vi "Main.vi"() -> ()   [LabVIEW 2013]
doc: "This Continuous Measurement sample project is based on the Queued Message Handler template.\n\nThe Event Handling Loop generates messages based on user interface actions.\n\nThe Message Handling Loop processes messages generated by the Event Handling Loop, or by other messages. There are also Acquisition and Logging message handling loop subVIs, and a chart updating loop."
uses:
  Settings/Settings.ctl
  Logging/Logging Configuration.ctl
  Piezo/Hardware Configuration.ctl
  Capacitive/Hardware Configuration.ctl
  Acquisition/Hardware Configuration.ctl
  Acquisition/Counter Configuration.ctl
  ADC/ADC Configuration.ctl
  controls/UI Data.ctl
  controls/UI State.ctl
  support/Message Queue/Enqueue Message (Single).vi
  <vilib>/measure/madcrms.llb/Averaged DC-RMS for 1 Chan.vi
  <vilib>/Utility/error.llb/Error Cluster From Error Code.vi
  <vilib>/ErrorRing/Error Ring.xnode
  Acquisition/Acquisition.lvlib
  Logging/Logging.lvlib
  Settings/Settings.lvlib
  support/User Event - Stop/User Event - Stop.lvlib
  support/Message Queue/Message Queue.lvlib
  <vilib>/ptbypt/NI_PtbyPt.lvlib
  Piezo/Piezo.lvlib
  Feedback/Feedback.lvlib
  <vilib>/measure/NI_MAPro.lvlib
  XY/XY.lvlib
  support/Data Notifiers/Data Notifiers.lvlib
  Capacitive/Capacitive.lvlib
  Automation/Automation.lvlib
panel:
  in  "Max. Samp":i32=1000000 format="%^#.2e"
  in  "Abort":bool
  out "Auto Status":string
  out "Status 2":bool
  out "Waveform Chart 2":dbl(graph)
  out "mean":dbl format="%0.2f"
  out "Error":dbl(knob) scale=-300.0..300.0
  in  "Channel":i32(ring) items=["0", "1", "2", "3", "off"]
  in  "Red":i32(ring) items=["0", "1", "2", "3", "off"]
  in  "Blue":i32(ring) items=["0", "1", "2", "3", "off"]
  out "Sample Rate (s/s)":i32
  out "Waveform Chart":waveform(dbl)[](graph)
  in  "Start Z scan":bool
  in  "Enable Piezo":bool
  out "Path":path
  in  "Filename":string
  out "Data Source":string="Counter (APD)"
  in  "Feedback Settings":T1={"Setpoint (cnt)"=10.999878508704048, "Refresh Time (s)"=1.0, "K_p (nm/cnt)"=50.0, "Averaging Time"=1.0, "T_i (s)"=0.3, "T_d (s)"=1.0, "Error Signal Source"=1} {"Error Signal Source" items=["APD Signal", "Capacitive"]}
  in  "Scan!":bool
  in  "Auto \nFB On":bool
  out "Control Status":string
  in  "Averaging Time (s)":dbl=3.0
  in  "Average and send\nto Setpoint":bool
  out "average":dbl
  out "Cap Readout":sgl
  out "Cap Status":string
  in  "Enable Sensor":bool
  out "Status 4":string
  in  "initialize":bool
  in  "PSD points":i32=1000
  out "Status 3":string
  out "Y":sgl
  out "X":sgl
  in  "Next Button":bool
  in  "Up Button":bool
  in  "Down Button":bool
  in  "Previous Button":bool
  in  "Jog Speed":u16(ring) items=["0", "1", "2", "3"]
  in  "Enable XY":bool
  out "Status":bool
  in  "Enable Feedback!":bool
  in  "Scan Settings":T2={"Dwell Time (s)"=1.0, "Max Height"=10.0, "Min Height"=9.0, "Step Size (um)"=0.01}
  in  "Start Saving":bool
  out "PiezoPosition":sgl
  out "Scan Duration: (s)":dbl
  in  "Do move":bool
  in  "Move to (um)":sgl
  out "PSD":cluster{"t":dbl, dbl, "Power Spectrum":dbl[]}(graph)
  out "Data":waveform(dbl)[](graph)
  in  "Settings":bool
  in  "Start":bool
  in  "Stop":bool
  out "Status":string
  in  "Exit":bool
  # "Recording"
  # "Position Control"
  # "Acquisition"
  # "Automation"
  # "Piezo Controller"
  # "X-Y Stage"
  # "Displacement Sensor"
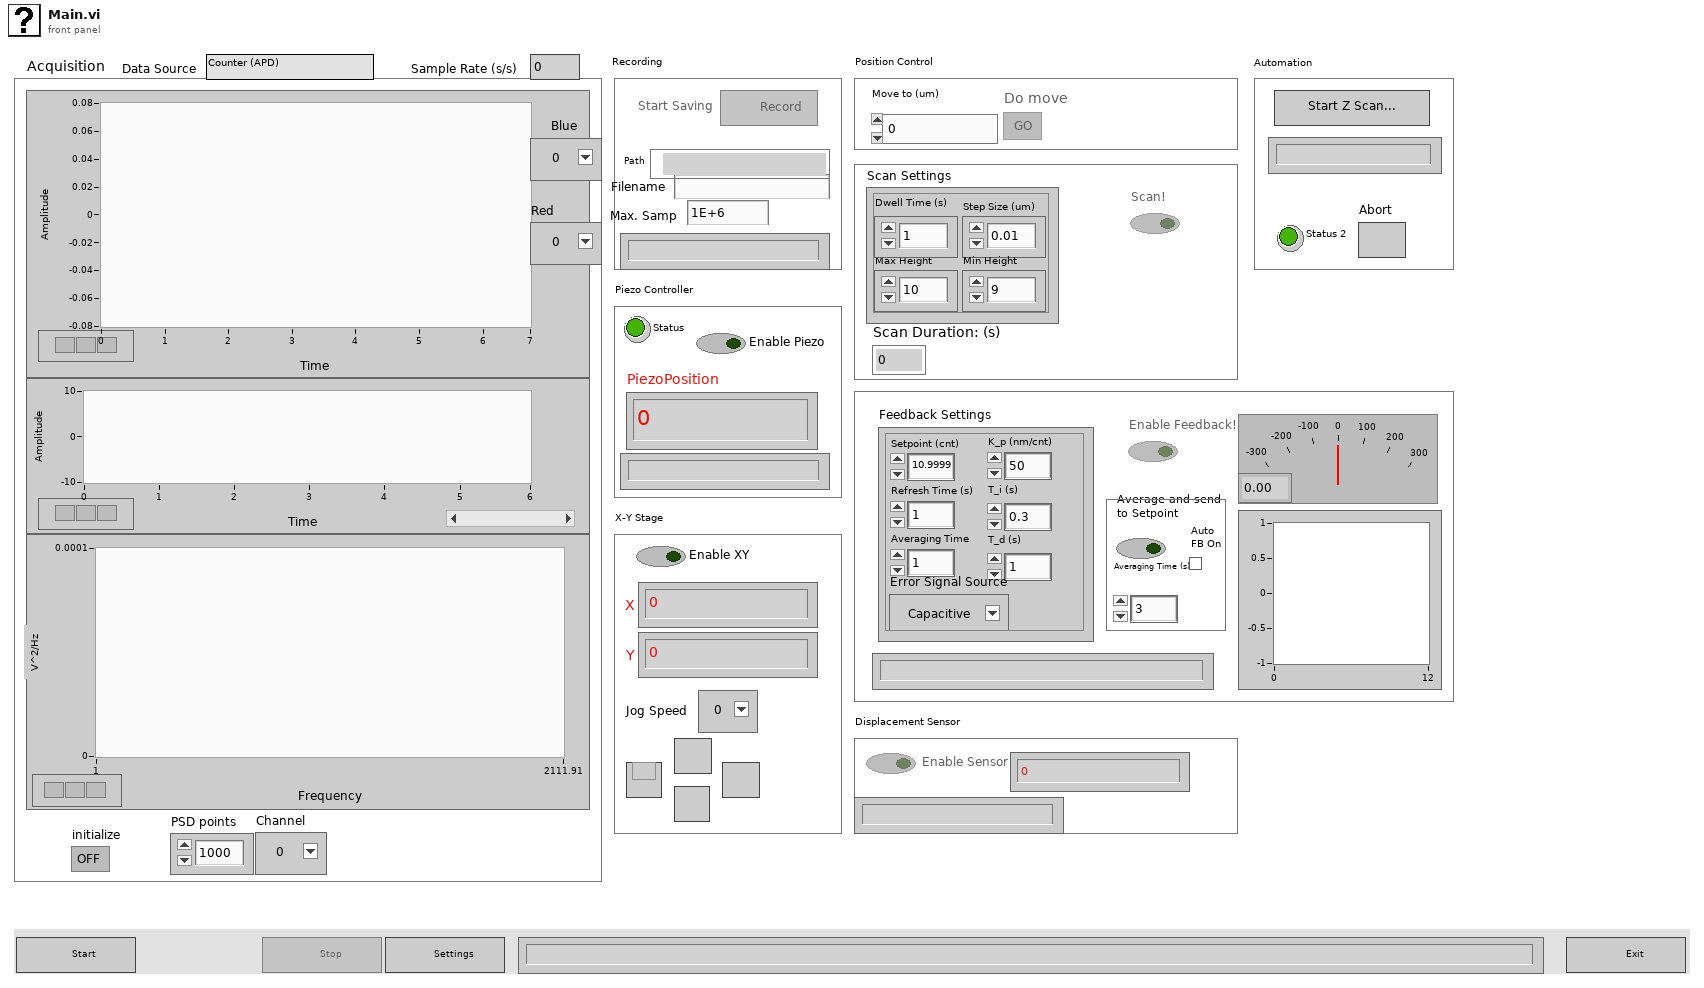
[diagram p1: front panel]
types:
  T1 = cluster{"Setpoint (cnt)":dbl, "Refresh Time (s)":dbl, "K_p (nm/cnt)":dbl, "Averaging Time":dbl, "T_i (s)":dbl, "T_d (s)":dbl, "Error Signal Source":u16}
  T2 = cluster{"Dwell Time (s)":dbl, "Max Height":dbl, "Min Height":dbl, "Step Size (um)":dbl}
  T3 = typedef "UI State.ctl" = cluster{"UI State":enum16{"Idle", "Acquiring and Logging", "Waiting for Exit", "Waiting for Stop"}, "Acq On":bool, "Log On":bool, "Piezo On":bool, "XY On":bool, "Cap On":bool}
  T4 = typedef "UI Data.ctl" = cluster{"Start Ref":refnum<vi>, "Trigger Ref":refnum<vi>, "Stop Ref":refnum<vi>, "Settings Ref":refnum<vi>, "Status Ref":refnum<vi>, "Exit Ref":refnum<vi>, "Data Ref":refnum<vi>, "Record Ref":refnum<vi>, "Scan Ref":refnum<vi>, "Feedback Ref":refnum<vi>, "Enable Sensor Ref":refnum<vi>, "Enable XY Ref":refnum<vi>, "Do move ref":refnum<vi>, "Enable Piezo":refnum<vi>}
  T5 = typedef "Settings.lvlib/Settings.ctl" = cluster{"Logging Configuration":T6, "Piezo Config":T7, "Capacitive Config":T8, "Hardware Config":T9}
  T6 = typedef "Logging.lvlib/Logging Configuration.ctl" = cluster{"Log File Base Path":path, "Max Samples":u32, "File Refnum":refnum<file>, "Log Piezo":bool, "Piezo File Refnum":refnum<file>, "Log Capacitive":bool, "Cap File Refnum":refnum<file>, "Filename":string, "Path where to save":path}
  T7 = typedef "Piezo.lvlib/Hardware Configuration.ctl" = cluster{"Piezo Serial Number":i32, "MG17Piezo":refnum<k7>, "Setpoint (um)":sgl}
  T8 = typedef "Capacitive.lvlib/Hardware Configuration.ctl" = cluster{"IP Address":string, "Handle":u32, "Refresh Time (ms)":dbl}
  T9 = typedef "Acquisition.lvlib/Hardware Configuration.ctl" = cluster{"Data Source":u16, "Counter Configuration":T10, "ADC Configuration":T11}
  T10 = typedef "Acquisition.lvlib/Counter Configuration.ctl" = cluster{"DAQmx Task":refnum<k21>, "Counter(s)":tag, "samples per readout":i32}
  T11 = typedef "Acquisition.lvlib/ADC Configuration.ctl" = cluster{"DAQmx Task":refnum<k21>, "Channel(s)":tag, "samples per readout":i32, "Sample Rate (s/s)":i32, "Max Voltage":dbl, "Min Voltage":dbl}
  T12 = typedef "Data Notifiers.lvlib/All Data Notifiers.ctl" = cluster{"APD Data Notifier":refnum<notifier>, "Piezo Readout Notifier":refnum<notifier>, "XY Readout Notifier":refnum<notifier>, "Capacitive Readout Notifier":refnum<notifier>, "Error Signal Notifier":refnum<notifier>}
  T13 = typedef "Message Queue.lvlib/All Message Queues.ctl" = cluster{"UI":refnum<queue>, "Acquisition":refnum<queue>, "Logging":refnum<queue>, "Piezo":refnum<queue>, "Feedback":refnum<queue>, "XY":refnum<queue>, "Capacitive":refnum<queue>, "Automation":refnum<queue>}
  T14 = enum16{"Idle", "Acquiring and Logging", "Waiting for Exit", "Waiting for Stop"}
  T15 = enum8{"Enabled", "Disabled", "Disabled and Grayed Out"}
  T16 = cluster{"Averaging Time (s)\n":dbl, "Error Signal Source":u16}
  T17 = cluster{"Value":bool, "Filename":string, "Max. Samp":i32}
  T18 = typedef "Automation.lvlib/Zscan Settings.ctl" = cluster{"Heights":dbl[], "Seconds per height":i32, "First Data Index":i32}
  T19 = typedef "XY.lvlib/XY Display.ctl" = cluster{"X Position":sgl, "Y Position":sgl}
  T20 = typedef "Acquisition.lvlib/APD Notifier Cluster.ctl" = cluster{"data":dbl[][], "t0":i32}
  T21 = typedef "Piezo.lvlib/Piezo display.ctl" = cluster{"PiezoPosition":sgl, "Counter Time":i32}
  T22 = typedef "Control 3.ctl" = cluster{"Error signal":dbl[], "Setpoint":dbl, "Last average":dbl}
  T23 = typedef "Capacitive.lvlib/Capacitive Signal Cluster.ctl" = cluster{"Readout":sgl, "Time":i32, "Temperature":dbl}
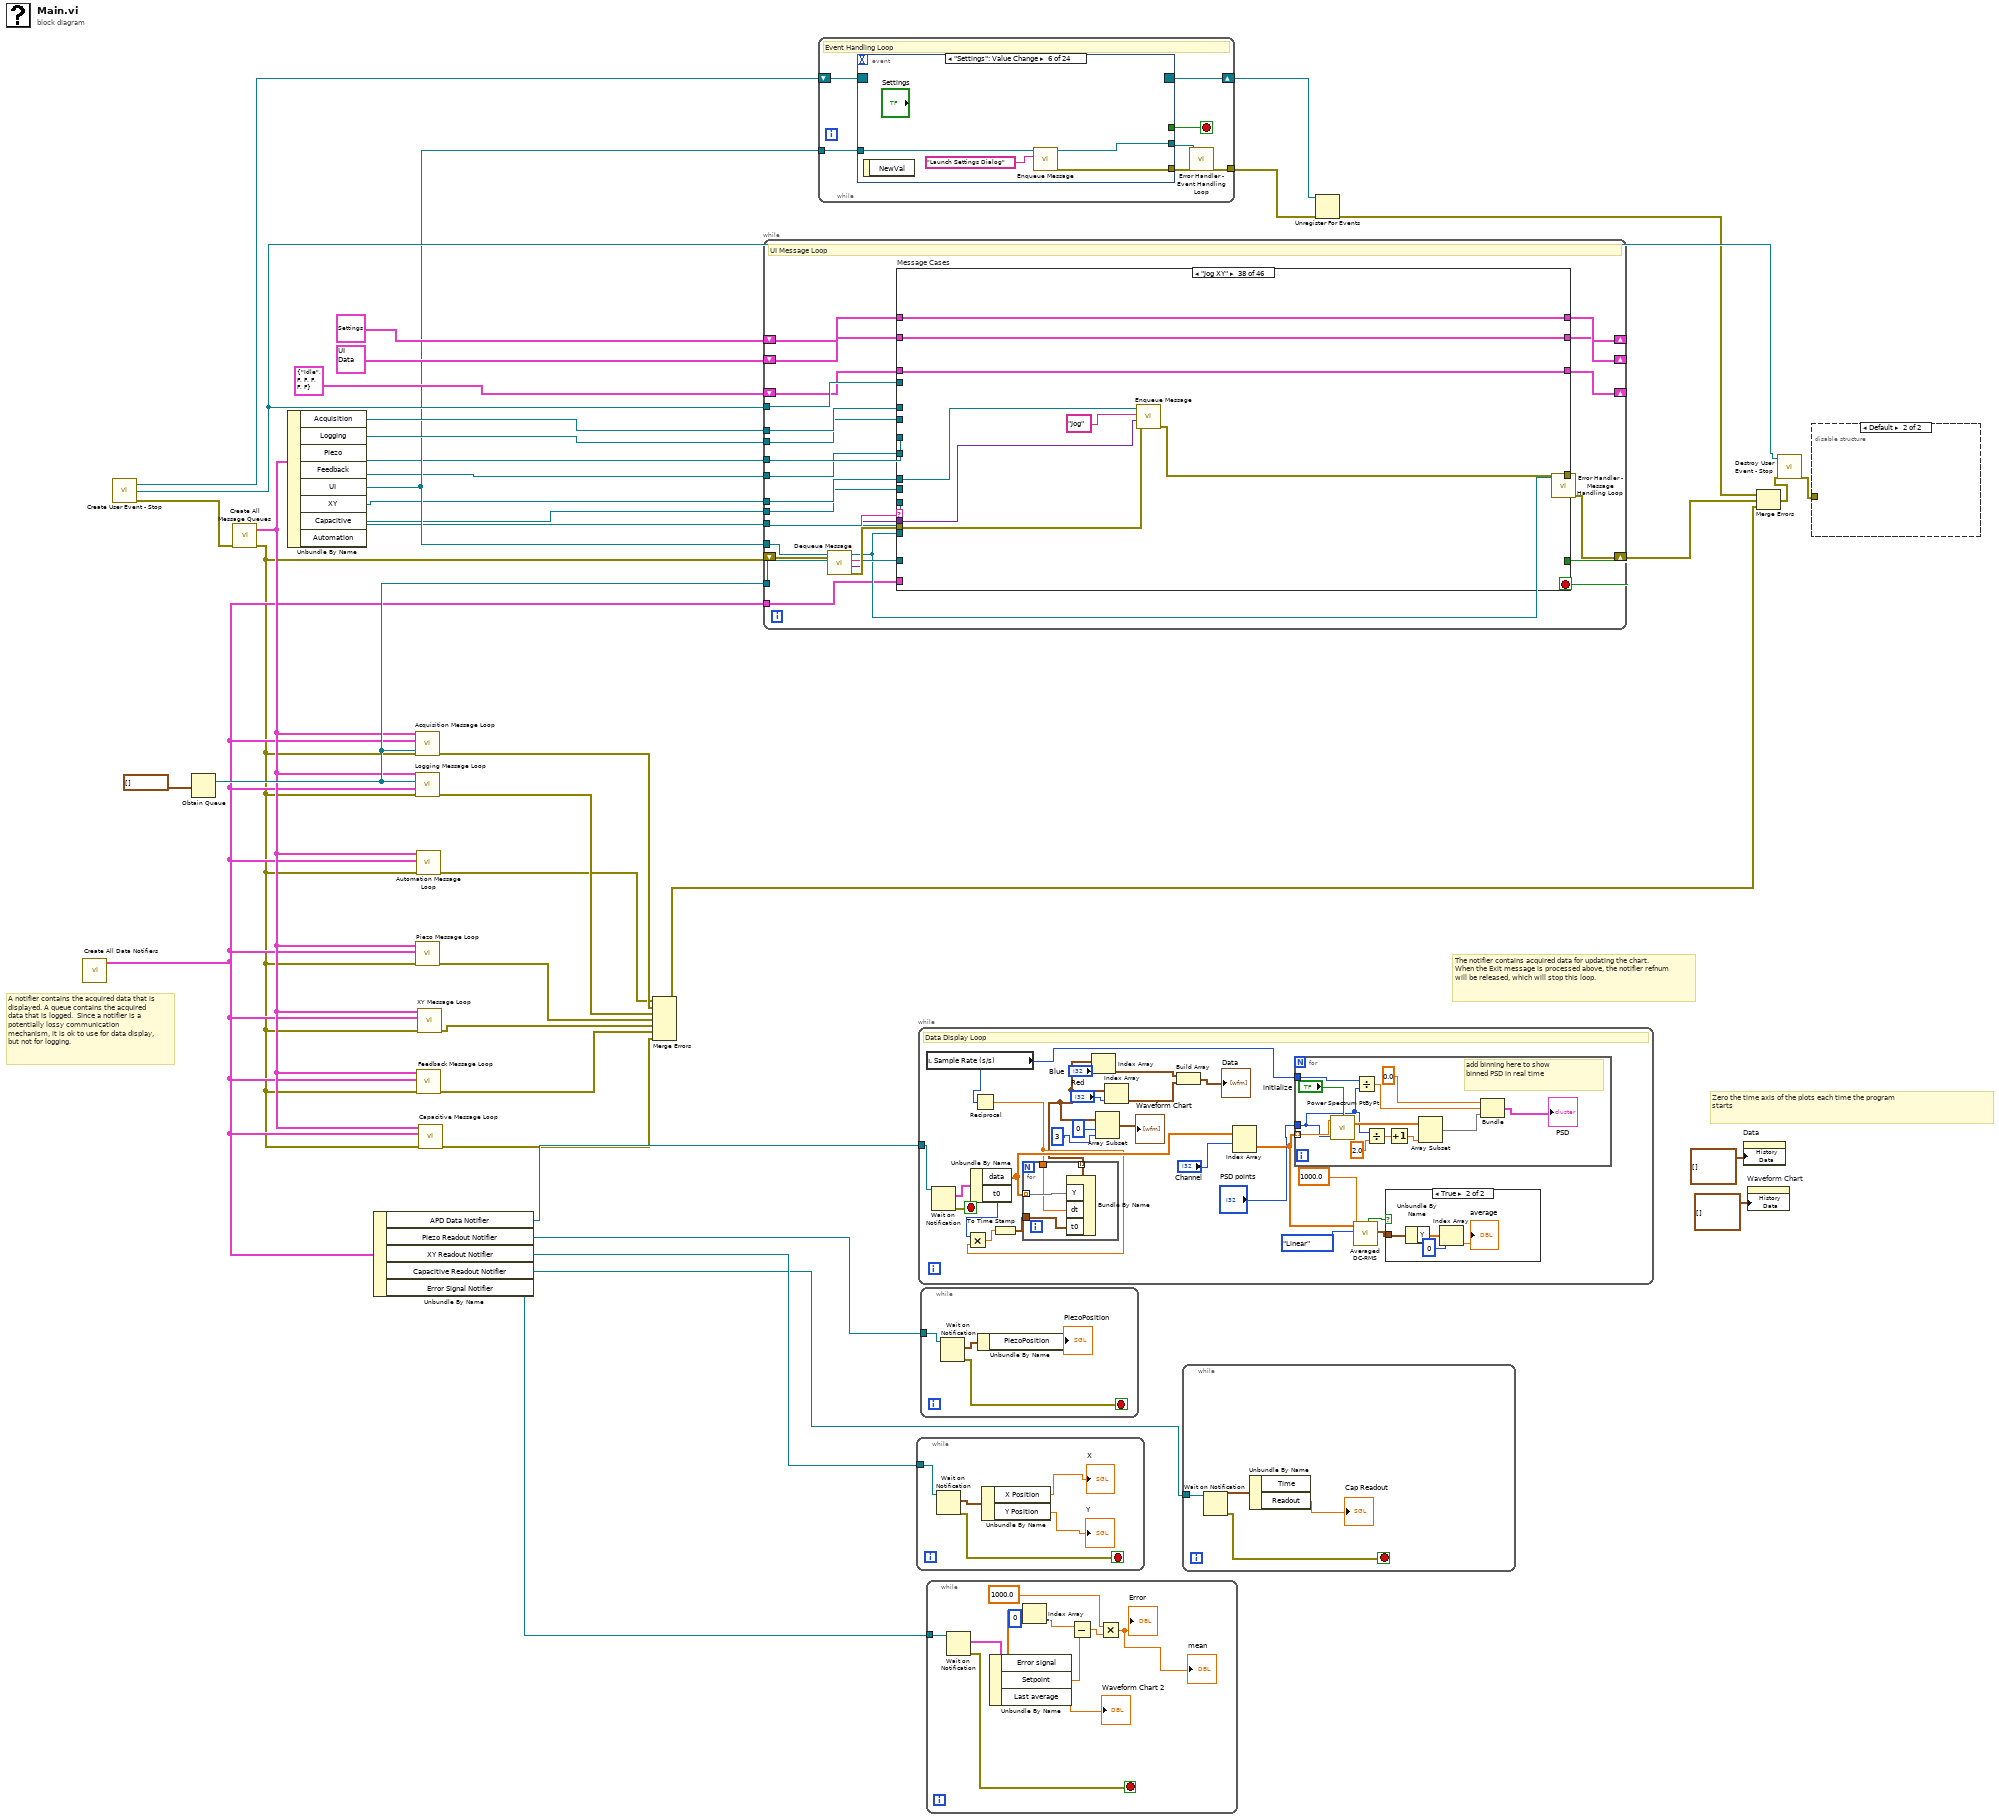
[diagram p0: block diagram]
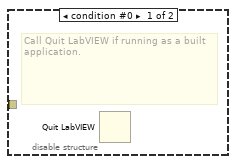
[diagram p2: hidden frame]
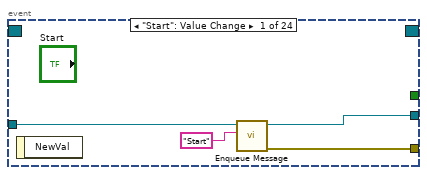
[diagram p4: hidden frame]
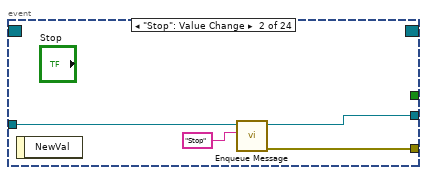
[diagram p5: hidden frame]
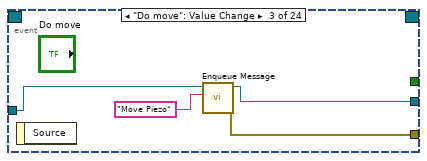
[diagram p6: hidden frame]
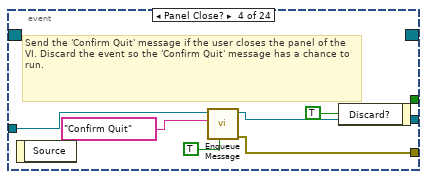
[diagram p7: hidden frame]
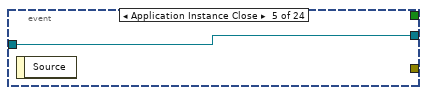
[diagram p8: hidden frame]
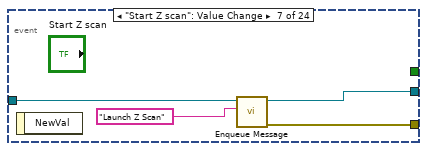
[diagram p9: hidden frame]
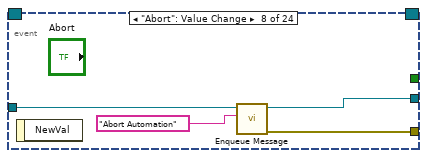
[diagram p10: hidden frame]
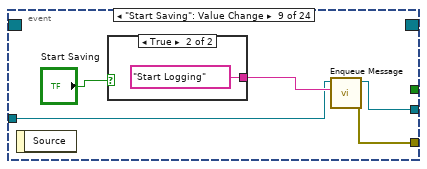
[diagram p11: hidden frame]
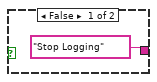
[diagram p12: hidden frame]
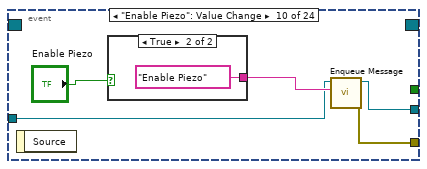
[diagram p13: hidden frame]
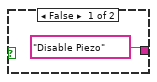
[diagram p14: hidden frame]
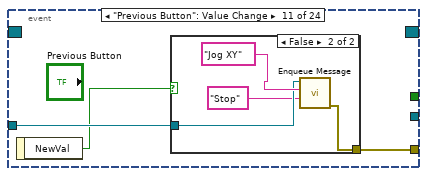
[diagram p15: hidden frame]
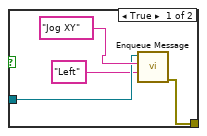
[diagram p16: hidden frame]
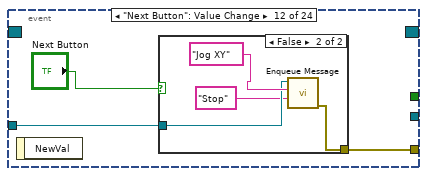
[diagram p17: hidden frame]
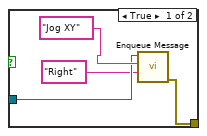
[diagram p18: hidden frame]
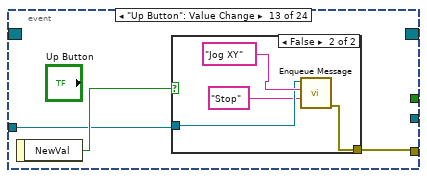
[diagram p19: hidden frame]
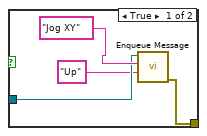
[diagram p20: hidden frame]
diagram:
  # "Zero the time axis of the plots each time the program \nstarts"
  # "A notifier contains the acquired data that is displayed. A queue contains the acquired data that is logged.  Since a notifier is a potentially lossy communication mechanism, it is ok to use for data display, but not for logging."
  # "The notifier contains acquired data for updating the chart. When the Exit message is processed above, the notifier refnum will be released, which will stop this loop."
  n1 = call "Create All Data Notifiers.vi"() -> ("Initialized Data Notifiers"=w3:T12)  [unwired: 11 in]
  n2 = call "Create User Event - Stop.vi"() -> ("error out"=w35:errorcluster, "User Event - Stop"=w36:refnum<user-event>, "Stop Event Registration Refnum"=w37:refnum<event-registration>)  [unwired: 9 in]
  n3 = Obtain Queue(element data type=waveform(dbl)[] []) -> (queue out=w27:refnum<queue>)  [unwired: 4 in, 2 out]
  n4 = call "Create All Message Queues.vi"("error in (no error)"=w35) -> ("error out"=w2:errorcluster, "Message Queues out"=w4:T13)  [unwired: 9 in]
  n5 = Unbundle By Name(w4) -> ("Acquisition"=w30:refnum<queue>, "Logging"=w29:refnum<queue>, "Piezo"=w23:refnum<queue>, "Feedback"=w22:refnum<queue>, "UI"=w24:refnum<queue>, "XY"=w21:refnum<queue>, "Capacitive"=w17:refnum<queue>, "Automation"=w5:refnum<queue>)
  n6 = Unbundle By Name(w3) -> ("APD Data Notifier"=w20:refnum<notifier>, "Piezo Readout Notifier"=w19:refnum<notifier>, "XY Readout Notifier"=w18:refnum<notifier>, "Capacitive Readout Notifier"=w9:refnum<notifier>, "Error Signal Notifier"=w6:refnum<notifier>)
  n7 = call "Acquisition Message Loop.vi"("error in (no error)"=w2, "Data Queue"=w27, "Data Notifiers"=w3, "Message Queues"=w4) -> ("error out"=w13:errorcluster)  [unwired: 7 in]
  n8 = call "Logging Message Loop.vi"("error in (no error)"=w2, "Data Notifiers"=w3, "Data Queue"=w27, "Message Queues"=w4) -> ("error out"=w14:errorcluster)  [unwired: 7 in]
  n9 = call "Piezo Message Loop.vi"("error in (no error)"=w2, "Data Notifiers"=w3, "Message Queues"=w4) -> ("error out"=w15:errorcluster)  [unwired: 8 in]
  n10 = call "Automation Message Loop.vi"("error in (no error)"=w2, "Data Notifiers"=w3, "Message Queues"=w4) -> ("error out"=w1:errorcluster)  [unwired: 8 in]
  n11 = call "Feedback Message Loop.vi"("error in (no error)"=w2, "Data Notifiers"=w3, "Message Queues"=w4) -> ("error out"=w12:errorcluster)  [unwired: 8 in]
  n12 = call "XY Message Loop.vi"("error in (no error)"=w2, "Data Notifiers"=w3, "Message Queues"=w4) -> ("error out"=w16:errorcluster)  [unwired: 8 in]
  n13 = call "Capacitive Message Loop.vi"("error in (no error)"=w2, "Data Notifiers"=w3, "Message Queues"=w4) -> ("error out"=w11:errorcluster)  [unwired: 8 in]
  n14 = Merge Errors(w1, w13, w14, w15, w16, w12, w11) -> (w10:errorcluster)
  n15 = while {
    tunnel: w24 -> [w59]
    tunnel: w36 -> [w64]
    shift-right: [w50] -> w40
    shift-left: w2 -> [w63]
    shift-right: [w58] -> _
    shift-left: T5 {"Logging Configuration"={"Log File Base Path"=path "", "Max Samples"=0, "File Refnum"=refnum, "Log Piezo"=FALSE, "Piezo File Refnum"=refnum, "Log Capacitive"=FALSE, "Cap File Refnum"=refnum, "Filename"="", "Path where to save"=path ""}, "Piezo Config"={"Piezo Serial Number"=0, "MG17Piezo"=refnum, "Setpoint (um)"=0.0}, "Capacitive Config"={"IP Address"="", "Handle"=0, "Refresh Time (ms)"=0.0}, "Hardware Config"={"Data Source"=0, "Counter Configuration"={"DAQmx Task"="", "Counter(s)"="", "samples per readout"=0}, "ADC Configuration"={"DAQmx Task"="", "Channel(s)"="", "samples per readout"=0, "Sample Rate (s/s)"=0, "Max Voltage"=0.0, "Min Voltage"=0.0}}} ("Settings") -> [w57]
    shift-right: [w55] -> _
    shift-left: T4 {"Start Ref"=refnum, "Trigger Ref"=refnum, "Stop Ref"=refnum, "Settings Ref"=refnum, "Status Ref"=refnum, "Exit Ref"=refnum, "Data Ref"=refnum, "Record Ref"=refnum, "Scan Ref"=refnum, "Feedback Ref"=refnum, "Enable Sensor Ref"=refnum, "Enable XY Ref"=refnum, "Do move ref"=refnum, "Enable Piezo"=refnum} ("Measurement UI Controls") -> [w56]
    tunnel: w30 -> [w54]
    tunnel: w29 -> [w53]
    tunnel: w27 -> [w52]
    shift-right: [w47] -> _
    shift-left: T3 {"UI State"=enum."Idle", "Acq On"=FALSE, "Log On"=FALSE, "Piezo On"=FALSE, "XY On"=FALSE, "Cap On"=FALSE} ("UI State") -> [w48]
    tunnel: w23 -> [w46]
    tunnel: w22 -> [w45]
    tunnel: w21 -> [w44]
    tunnel: w3 -> [w43]
    tunnel: w17 -> [w42]
    tunnel: w5 -> [w41]
    stop <- w65 stop-if-true
    # "UI Message Loop"
    n16 = call "Dequeue Message.vi"("error in (no error)"=w63, "Message Queue"=w59) -> ("error out"=w62:errorcluster, "Message Data"=w60:variant, "Message"=w61:string, "dup Message Queue"=w49:refnum<queue>)  [unwired: 6 in]
    n17 = case "Message Cases" shown="\"Jog XY\"" w61 {
      selector: w61 -> [_ _ _ _ _ _ _ _ _ _ _ _ _ _ _ _ _ _ _ _ _ _ _ _ _ _ _ _ _ _ _ _ _ _ _ _ _ _ _ _ _ _ _ _ _ w807]
      tunnel: w49 -> [w70 _ _ _ _ _ _ _ w282 w317 w329 w351 w369 w388 w411 _ w455 w470 w482 w520 _ _ _ _ _ _ _ _ _ _ _ _ _ _ _ _ _ _ _ _ _ _ _ w773 w793 _]
      tunnel: w62 -> [w69 w103 w114 w128 w139 w153 w167 w186 w281 w316 w327 w349 w367 w386 w410 w444 w457 w474 w481 w525 w535 w540 w547 w555 w567 w574 w589 w605 w613 w624 w640 w649 w665 w672 w680 w696 w707 w713 w722 w730 w738 w750 w761 w775 w795 _]
      tunnel: [w76 w103 w115 w129 w140 w154 w168 w187 w283 w304 w328 w350 w368 w387 w407 w447 w452 w465 w480 w526 w534 w539 w553 w561 w566 w580 w583 w611 w619 w630 w644 w655 w669 w677 w686 w700 w711 w712 w721 w735 w743 w754 w765 w776 w796 w808] -> w51
      tunnel: [_ _ _ _ _ _ _ _ _ _ _ _ _ _ _ _ _ _ _ TRUE _ _ _ _ _ _ _ _ _ _ _ _ _ _ _ _ _ _ _ _ _ _ _ _ _ _] -> w65
      tunnel: w60 -> [_ _ w113 w127 w138 w152 w166 w185 _ _ _ _ _ _ _ _ _ w473 _ _ _ _ _ _ _ _ w588 _ _ w631 _ _ _ _ _ _ _ w716 w723 _ _ _ _ _ _ _]
      tunnel: w64 -> [_ _ _ _ _ _ _ _ _ _ _ _ _ _ _ _ _ _ _ w524 _ _ _ _ _ _ _ _ _ _ _ _ _ _ _ _ _ _ _ _ _ _ _ _ _ _]
      tunnel: [w79 w102 w110 w124 w135 w149 w163 w183 w280 w315 w335 w356 w375 w394 w417 w431 w454 w476 w484 w522 w533 w543 w552 w560 w572 w579 w592 w610 w618 w634 w643 w654 w668 w676 w685 w699 w710 w719 w727 w734 w742 w753 w764 w778 w798 w810] -> w58
      tunnel: w57 -> [w80 w102 w110 w124 w135 w149 w163 w183 w280 w315 w335 w356 w375 w394 w417 w431 w458 w476 w484 w522 w533 w543 w552 w560 w572 w579 w592 w610 w618 w634 w643 w654 w668 w676 w685 w699 w710 w719 w727 w734 w742 w753 w764 w778 w798 w810]
      tunnel: w56 -> [w72 w101 w109 w123 w131 w145 w162 w182 w262 w297 w334 w348 w374 w393 w416 w443 w451 w475 w483 w521 w532 w542 w551 w559 w571 w578 w591 w609 w617 w633 w636 w651 w663 w675 w684 w692 w703 w718 w726 w733 w741 w747 w758 w777 w797 w809]
      tunnel: [w72 w100 w109 w123 w131 w145 w162 w182 w262 w297 w334 w348 w374 w393 w416 w443 w451 w475 w483 w521 w532 w542 w551 w559 w571 w578 w591 w609 w617 w633 w636 w651 w663 w675 w684 w692 w703 w718 w726 w733 w741 w747 w758 w777 w797 w809] -> w55
      tunnel: w54 -> [_ _ _ _ _ _ _ _ w273 w293 _ _ _ _ _ w442 _ _ _ w513 _ _ _ _ _ _ _ _ _ _ _ _ _ _ _ _ _ _ _ _ _ _ _ _ _ _]
      tunnel: w53 -> [_ _ _ _ _ _ _ _ _ w292 _ _ _ _ _ w441 _ _ _ w512 _ _ _ _ _ _ _ w606 w614 _ _ _ _ _ _ _ _ _ _ _ _ _ _ _ _ _]
      tunnel: w52 -> [_ _ _ _ _ _ _ _ _ _ _ _ _ _ _ _ _ _ _ w519 _ _ _ _ _ _ _ _ _ _ _ _ _ _ _ _ _ _ _ _ _ _ _ _ _ _]
      tunnel: w48 -> [_ _ w104 w121 w134 w148 w161 w181 _ w305 w332 w354 w372 w391 w414 w440 w450 w464 w478 _ w531 w536 w550 w558 w570 w577 w590 w608 w616 w623 w642 w653 w667 w674 w683 w698 w709 w714 w720 w732 w740 w752 w763 w774 w794 w806]
      tunnel: [T3 {"UI State"=enum."Idle", "Acq On"=FALSE, "Log On"=FALSE, "Piezo On"=FALSE, "XY On"=FALSE, "Cap On"=FALSE} ("UI State") T3 {"UI State"=enum."Idle", "Acq On"=FALSE, "Log On"=FALSE, "Piezo On"=FALSE, "XY On"=FALSE, "Cap On"=FALSE} ("UI State") w104 w121 w134 w148 w161 w181 T3 {"UI State"=enum."Idle", "Acq On"=TRUE, "Log On"=TRUE, "Piezo On"=TRUE, "XY On"=FALSE, "Cap On"=FALSE} ("UI State") w307 w332 w354 w372 w391 w414 w440 w450 w464 w479 T3 {"UI State"=enum."Idle", "Acq On"=FALSE, "Log On"=FALSE, "Piezo On"=FALSE, "XY On"=FALSE, "Cap On"=FALSE} ("UI State") w531 w536 w550 w558 w570 w577 w590 w608 w616 w623 w642 w653 w667 w674 w683 w698 w709 w714 w720 w732 w740 w752 w763 w774 w794 w806] -> w47
      tunnel: w46 -> [_ _ _ _ _ _ _ _ w271 w291 _ _ _ _ _ _ _ _ _ w511 _ _ _ _ _ _ _ _ _ _ _ _ _ _ _ _ _ _ _ _ _ w748 w759 _ _ _]
      tunnel: w45 -> [_ _ _ _ _ _ _ _ w267 w290 _ _ _ _ _ _ _ _ _ w510 _ w538 w548 w556 w568 w575 _ _ _ _ w637 _ _ w670 w678 _ _ _ _ _ _ _ _ _ _ _]
      tunnel: w44 -> [_ _ _ _ _ _ _ _ _ w289 _ _ _ _ _ _ _ _ _ w509 _ _ _ _ _ _ _ _ _ _ _ _ _ _ _ w694 w705 w717 w724 _ _ _ _ _ _ _]
      tunnel: w43 -> [_ _ _ _ _ _ _ _ _ _ _ _ _ _ _ _ _ _ _ w516 _ _ _ _ _ _ _ _ _ _ _ _ _ _ _ _ _ _ _ _ _ _ _ _ _ _]
      tunnel: w42 -> [_ _ _ _ _ _ _ _ w264 w288 _ _ _ _ _ w439 _ _ _ w507 _ _ _ _ _ _ _ _ _ _ _ _ _ _ _ _ _ _ _ w728 w736 _ _ _ _ _]
      tunnel: w41 -> [_ _ _ _ _ _ _ _ _ w287 _ _ _ _ _ _ _ _ _ w506 _ _ _ _ _ _ _ _ _ _ _ w650 w662 _ _ _ _ _ _ _ _ _ _ _ _ _]
      frame "Initialize" {
        # "Initialize - Get configuration settings, then message the UI to initialize, and broadcast the settings to the other message loops."
        n18 = call "Load Settings from XML.vi"("Settings in"=w80) -> ("Settings out"=w79:T5)  [unwired: 9 in, 1 out]
        n19 = call-poly "Enqueue Message.vi"("error in (no error)"=w69, "Message"="Init UI Refs", "Message Queue"=w70) -> ("error out"=w67:errorcluster, "dup Message Queue"=w68:refnum<queue>)  [unwired: 7 in]
        n20 = call-poly "Enqueue Message.vi"("error in (no error)"=w67, "Message"="Broadcast Settings", "Message Queue"=w68) -> ("error out"=w78:errorcluster, "dup Message Queue"=w77:refnum<queue>)  [unwired: 7 in]
        n21 = call-poly "Enqueue Message.vi"("error in (no error)"=w78, "Message Data"="Ready..." ("Ready..."), "Message"="Update Status", "Message Queue"=w77) -> ("error out"=w76:errorcluster)  [unwired: 6 in, 1 out]
      }
      frame "Init UI Refs" {
        # "Enable: Start, Exit, Settings\nDisable: Stop"
        # "Init UI Refs - Store control references for UI controls.  Also enable/disable controls appropriately."
        n22 = control-ref of="Data"() -> (w96:refnum<vi>)
        n23 = control-ref of="Exit"() -> (w91:refnum<vi>)
        n24 = control-ref of="Start"() -> (w95:refnum<vi>)
        n25 = control-ref of="Stop"() -> (w90:refnum<vi>)
        n26 = control-ref of="Settings"() -> (w92:refnum<vi>)
        n27 = control-ref of="Status"() -> (w97:refnum<vi>)
        n28 = control-ref of="Scan!"() -> (w86:refnum<vi>)
        n29 = control-ref of="Start Saving"() -> (w87:refnum<vi>)
        n30 = control-ref of="Do move"() -> (w83:refnum<vi>)
        n31 = control-ref of="Enable Piezo"() -> (w81:refnum<vi>)
        n32 = control-ref of="Enable Sensor"() -> (w84:refnum<vi>)
        n33 = control-ref of="Enable XY"() -> (w82:refnum<vi>)
        n34 = control-ref of="Enable Feedback!"() -> (w85:refnum<vi>)
        n35 = Build Array(w82, w91, w92, w95) -> (w94:refnum<vi>[])
        n36 = call "Set Enable State on Multiple Controls.vi"("Enable?"=TRUE, "Controls"=w94) -> ()  [unwired: 10 in]
        n37 = Build Array(w81, w83, w84, w85, w86, w87, w90) -> (w89:refnum<vi>[])
        n38 = call "Set Enable State on Multiple Controls.vi"("Enable?"=FALSE, "Controls"=w89) -> ()  [unwired: 10 in]
        n39 = Bundle By Name(cluster=w101, "Start Ref"=w95, "Stop Ref"=w90, "Settings Ref"=w92, "Status Ref"=w97, "Exit Ref"=w91, "Data Ref"=w96, "Record Ref"=w87, "Scan Ref"=w86, "Feedback Ref"=w85, "Enable Sensor Ref"=w84, "Enable XY Ref"=w82, "Do move ref"=w83, "Enable Piezo"=w81) -> (w100:T4)
        n40 = property class="VI"("Front Panel.Closeable"=TRUE ("Front Panel Window:Closeable")) -> ()  [unwired: 2 in, 2 out]
      }
      frame "Update Status" {
        # "Update Display - Convert the message data to a string to display in the Status indicator."
        n41 = Variant To Data(error in=w114, type="", Variant=w113) -> (data=w106:string, error out=w111:errorcluster)
        "Status" <- w106
        n42 = Unbundle By Name(w109) -> ("Trigger Ref"=w105:refnum<vi>, "Stop Ref"=w108:refnum<vi>)
        n43 = property class="Bool"(reference=w108) -> ("DisabledEnum"=w107:T15)  [unwired: 1 in, 2 out]
        n44 = case shown="\"Enabled\"" w107 {
          tunnel: w106 -> [w118 _]
          tunnel: w105 -> [w119 _]
          frame "Enabled" {
            # "Disable the Force Trigger only while we are logging."
            n45 = Build Array(w119) -> (w120:refnum<vi>[])
            n46 = Not Equal?(x="Logging" ("Logging"), y=w118) -> (x != y?=w116:bool)
            n47 = call "Set Enable State on Multiple Controls.vi"("Enable?"=w116, "Controls"=w120) -> ()  [unwired: 10 in]
          }
          frame "Disabled", Default {
          }
        }
        n48 = Merge Errors(w111) -> (w115:errorcluster)
      }
      frame "Log Status" {
        # "Update Display - Convert the message data to a string to display in the Status indicator."
        n49 = Variant To Data(error in=w128, type="", Variant=w127) -> (data=→"Status 3":string, error out=w125:errorcluster)
        n50 = Merge Errors(w125) -> (w129:errorcluster)
      }
      frame "Piezo Status" {
        # "Update Display - Convert the message data to a string to display in the Status indicator."
        n51 = Variant To Data(error in=w139, type="", Variant=w138) -> (data=w133:string, error out=w136:errorcluster)
        "Status 4" <- w133
        n52 = Unbundle By Name(w131) -> ("Enable Piezo"=w130:refnum<vi>)
        n53 = case shown="\"Stopped\", Default" w133 {
          tunnel: [w141 w143] -> w132
          tunnel: w130 -> [w142 w144]
          frame "Stopped", Default {
            w141 = FALSE
            n54 = property class="Bool"(reference=w142, "Value"=w141) -> ()  [unwired: 1 in, 2 out]
          }
          frame "Connected" {
            w143 = TRUE ("Status")
            n55 = property class="Bool"(reference=w144, "Value"=w143) -> ()  [unwired: 1 in, 2 out]
          }
        }
        "Status" <- w132
        n56 = Merge Errors(w136) -> (w140:errorcluster)
      }
      frame "Auto Status" {
        # "Update Display - Convert the message data to a string to display in the Status indicator."
        n57 = Variant To Data(error in=w153, type="", Variant=w152) -> (data=w147:string, error out=w150:errorcluster)
        "Auto Status" <- w147
        n58 = case shown="\"Stopped\"" w147 {
          tunnel: [FALSE TRUE ("Status") TRUE ("Status")] -> w146
          frame "Stopped" {
          }
          frame "Active" {
          }
          frame Default {
          }
        }
        "Status 2" <- w146
        n59 = Merge Errors(w150) -> (w154:errorcluster)
      }
      frame "Cap Status" {
        # "Update Display - Convert the message data to a string to display in the Status indicator."
        n60 = Variant To Data(error in=w167, type="", Variant=w166) -> (data=w160:string, error out=w164:errorcluster)
        "Cap Status" <- w160
        n61 = control-ref of="Enable Sensor"() -> (w159:refnum<vi>)
        n62 = case shown="\"Acquiring\"" w160 {
          tunnel: w159 -> [w170 w174]
          tunnel: [w171 w172] -> w158
          frame "Acquiring" {
            n63 = property class="Bool (strict)"(reference=w170, "Value"=TRUE) -> (error out=w171:errorcluster)  [unwired: 1 in, 1 out]
          }
          frame "Stopped", Default {
            n64 = property class="Bool (strict)"(reference=w174, "Value"=FALSE) -> (error out=w172:errorcluster)  [unwired: 1 in, 1 out]
          }
        }
        n65 = Merge Errors(w158, w164) -> (w168:errorcluster)
      }
      frame "Feedback Status" {
        # "Update Display - Convert the message data to a string to display in the Status indicator."
        n66 = Variant To Data(error in=w186, type="", Variant=w185) -> (data=w180:string, error out=w179:errorcluster)
        "Control Status" <- w180
        n67 = control-ref of="Average and send\nto Setpoint"() -> (w175:refnum<vi>)
        n68 = control-ref of="Enable Feedback!"() -> (w177:refnum<vi>)
        n69 = control-ref of="Scan!"() -> (w176:refnum<vi>)
        n70 = case shown="\"Feedback Started...\"" w180 {
          tunnel: w179 -> [w188 w194 w203 w209 w217 w226 w235 w238 w247]
          tunnel: [w188 w189 w195 w205 w215 w225 w233 w243 w251] -> w178
          tunnel: w177 -> [_ w193 w198 w208 w216 w220 w234 w244 w252]
          tunnel: w176 -> [_ w192 w202 _ w212 w222 w229 w240 w248]
          tunnel: w175 -> [_ _ w199 w204 w210 w219 w228 w241 w249]
          frame "False", Default {
          }
          frame "Averaging Started..." {
            w191 = T15."Disabled and Grayed Out" ("Disabled")
            # "Disable Scan and Feedback while averaging"
            n71 = property class="Bool (strict)"(reference=w193, error in=w194, "DisabledEnum"=w191) -> (error out=w190:errorcluster)  [unwired: 1 out]
            n72 = property class="Bool (strict)"(reference=w192, error in=w190, "DisabledEnum"=w191) -> (error out=w189:errorcluster)  [unwired: 1 out]
          }
          frame "Feedback Started..." {
            w201 = T15."Disabled and Grayed Out" ("Disabled")
            # "Disable Scan and Average while Feedback On"
            n73 = property class="Bool (strict)"(reference=w199, error in=w203, "DisabledEnum"=w201) -> (error out=w200:errorcluster)  [unwired: 1 out]
            n74 = property class="Bool (strict)"(reference=w202, error in=w200, "DisabledEnum"=w201) -> (error out=w196:errorcluster)  [unwired: 1 out]
            n75 = property class="Bool (strict)"(reference=w198, error in=w196, "Value"=TRUE) -> (error out=w195:errorcluster)  [unwired: 1 out]
          }
          frame "Scan Started..." {
            w207 = T15."Disabled and Grayed Out" ("Disabled")
            # "Disable Avg and Feedback while Scanning"
            n76 = property class="Bool (strict)"(reference=w208, error in=w209, "DisabledEnum"=w207) -> (error out=w206:errorcluster)  [unwired: 1 out]
            n77 = property class="Bool (strict)"(reference=w204, error in=w206, "DisabledEnum"=w207) -> (error out=w205:errorcluster)  [unwired: 1 out]
          }
          frame "Averaging stopped... Ready" {
            w211 = T15."Enabled" ("Disabled")
            # "Enable Scan and Feedback buttons once averaging stopped"
            n78 = property class="Bool (strict)"(reference=w210, error in=w217, "Value"=FALSE) -> (error out=w214:errorcluster)  [unwired: 1 out]
            n79 = property class="Bool (strict)"(reference=w212, error in=w214, "DisabledEnum"=w211) -> (error out=w213:errorcluster)  [unwired: 1 out]
            n80 = property class="Bool (strict)"(reference=w216, error in=w213, "DisabledEnum"=w211) -> (error out=w215:errorcluster)  [unwired: 1 out]
          }
          frame "Feedback Stopped... Ready" {
            w221 = T15."Enabled" ("Disabled")
            # "Enable Scan and Average buttons once Feedback stopped"
            n81 = property class="Bool (strict)"(reference=w220, error in=w226, "Value"=FALSE) -> (error out=w224:errorcluster)  [unwired: 1 out]
            n82 = property class="Bool (strict)"(reference=w222, error in=w224, "DisabledEnum"=w221) -> (error out=w223:errorcluster)  [unwired: 1 out]
            n83 = property class="Bool (strict)"(reference=w219, error in=w223, "DisabledEnum"=w221) -> (error out=w225:errorcluster)  [unwired: 1 out]
          }
          frame "Scan Stopped... Ready" {
            w230 = T15."Enabled" ("Disabled")
            # "Enable Scan and Feedback buttons once averaging stopped"
            n84 = property class="Bool (strict)"(reference=w229, error in=w235, "Value"=FALSE) -> (error out=w232:errorcluster)  [unwired: 1 out]
            n85 = property class="Bool (strict)"(reference=w228, error in=w232, "DisabledEnum"=w230) -> (error out=w231:errorcluster)  [unwired: 1 out]
            n86 = property class="Bool (strict)"(reference=w234, error in=w231, "DisabledEnum"=w230) -> (error out=w233:errorcluster)  [unwired: 1 out]
          }
          frame "Ready..." {
            w239 = T15."Enabled" ("Disabled")
            # "Make sure all are enabled at first, in case program crashed\nearlier"
            n87 = property class="Bool (strict)"(reference=w240, error in=w238, "DisabledEnum"=w239) -> (error out=w237:errorcluster)  [unwired: 1 out]
            n88 = property class="Bool (strict)"(reference=w241, error in=w237, "DisabledEnum"=w239) -> (error out=w242:errorcluster)  [unwired: 1 out]
            n89 = property class="Bool (strict)"(reference=w244, error in=w242, "DisabledEnum"=w239) -> (error out=w243:errorcluster)  [unwired: 1 out]
          }
          frame "Stopped" {
            w245 = FALSE ("Value")
            # "Turn off all buttons if program is stopped"
            n90 = property class="Bool (strict)"(reference=w248, error in=w247, "Value"=w245) -> (error out=w246:errorcluster)  [unwired: 1 out]
            n91 = property class="Bool (strict)"(reference=w249, error in=w246, "Value"=w245) -> (error out=w250:errorcluster)  [unwired: 1 out]
            n92 = property class="Bool (strict)"(reference=w252, error in=w250, "Value"=w245) -> (error out=w251:errorcluster)  [unwired: 1 out]
          }
        }
        n93 = Merge Errors(w178) -> (w187:errorcluster)
      }
      frame "Start" {
        w263 = "Start" ("Message")
        # "Message Acquisition and Logging loops to start"
        # "Start - Enable/Disable buttons appropriately for an acquisition that has started, and update status display."
        n94 = Unbundle By Name(w262) -> ("Enable XY Ref"=w255:refnum<vi>, "Start Ref"=w275:refnum<vi>, "Exit Ref"=w274:refnum<vi>, "Settings Ref"=w253:refnum<vi>)
        n95 = Build Array(w255, w275, w274, w253) -> (w276:refnum<vi>[])
        n96 = call-poly "Enqueue Message.vi"("error in (no error)"=w281, "Message Data"="Started" ("Waiting for trigger"), "Message"="Update Status", "Message Queue"=w282) -> ("error out"=w270:errorcluster)  [unwired: 6 in, 1 out]
        n97 = call "Set Enable State on Multiple Controls.vi"("Enable?"=FALSE, "Controls"=w276) -> ()  [unwired: 10 in]
        n98 = Unbundle By Name(w262) -> ("Stop Ref"=w259:refnum<vi>, "Record Ref"=w258:refnum<vi>, "Do move ref"=w257:refnum<vi>, "Enable Sensor Ref"=w256:refnum<vi>, "Enable Piezo"=w254:refnum<vi>)
        n99 = call-poly "Enqueue Message.vi"("error in (no error)"=w270, "Message"=w263, "Message Queue"=w271) -> ("error out"=w269:errorcluster)  [unwired: 7 in, 1 out]
        n100 = call-poly "Enqueue Message.vi"("error in (no error)"=w269, "Message"=w263, "Message Queue"=w273) -> ("error out"=w268:errorcluster)  [unwired: 7 in, 1 out]
        n101 = Build Array(w259, w258, w257, w256, w254) -> (w261:refnum<vi>[])
        n102 = call-poly "Enqueue Message.vi"("error in (no error)"=w268, "Message"=w263, "Message Queue"=w267) -> ("error out"=w266:errorcluster)  [unwired: 7 in, 1 out]
        n103 = call "Set Enable State on Multiple Controls.vi"("Enable?"=TRUE, "Controls"=w261) -> ()  [unwired: 10 in]
        n104 = call-poly "Enqueue Message.vi"("error in (no error)"=w266, "Message"=w263, "Message Queue"=w264) -> ("error out"=w265:errorcluster)  [unwired: 7 in, 1 out]
        n105 = Merge Errors(w265) -> (w283:errorcluster)
      }
      frame "Stop" {
        # "Message All loops to stop"
        # "Stop - Enable/Disable buttons appropriately for an acquisition that has stopped, and update status display."
        n106 = Build Array(w293, w292, w291, w290, w289, w288, w287) -> (w286:refnum<queue>[])
        n107 = Unbundle By Name(w297) -> ("Start Ref"=w310:refnum<vi>, "Exit Ref"=w309:refnum<vi>, "Settings Ref"=w308:refnum<vi>, "Enable XY Ref"=w294:refnum<vi>)
        n108 = Unbundle By Name(w305) -> ("UI State"=w306:T14)
        n109 = call-poly "Enqueue Message.vi"("error in (no error)"=w316, "Message Data"="Ready..." ("Ready..."), "Message"="Update Status", "Message Queue"=w317) -> ("error out"=w285:errorcluster)  [unwired: 6 in, 1 out]
        n110 = Build Array(w310, w309, w308, w294) -> (w311:refnum<vi>[])
        n111 = call "Set Enable State on Multiple Controls.vi"("Enable?"=TRUE, "Controls"=w311) -> ()  [unwired: 10 in]
        n112 = Unbundle By Name(w297) -> ("Stop Ref"=w301:refnum<vi>, "Record Ref"=w300:refnum<vi>, "Do move ref"=w299:refnum<vi>, "Enable Sensor Ref"=w298:refnum<vi>, "Scan Ref"=w296:refnum<vi>, "Feedback Ref"=w295:refnum<vi>)
        n113 = for {
          tunnel: w286 -> [w321] mode=indexing
          shift-right: [w318] -> w284
          shift-left: w285 -> [w319]
          n114 = call-poly "Enqueue Message.vi"("Priority Message? (F)"=TRUE, "error in (no error)"=w319, "Message"="Stop", "Message Queue"=w321) -> ("error out"=w318:errorcluster)  [unwired: 6 in, 1 out]
        }
        n115 = Build Array(w301, w300, w299, w298, w296, w295) -> (w303:refnum<vi>[])
        n116 = call "Set Enable State on Multiple Controls.vi"("Enable?"=FALSE, "Controls"=w303) -> ()  [unwired: 10 in]
        n117 = case shown="Default" w306 {
          tunnel: [w323 w326] -> w307
          tunnel: w305 -> [w324 w326]
          frame Default {
            n118 = Bundle By Name(cluster=w324, "UI State"=T14."Waiting for Stop") -> (w323:T3)
          }
          frame "Waiting for Exit" {
          }
        }
        n119 = Merge Errors(w284) -> (w304:errorcluster)
      }
      frame "Acquisition Stopped" {
        # "Logic for determining what action to take when the acquisition has stopped."
        n120 = Bundle By Name(cluster=w332, "Acq On"=FALSE) -> (w331:T3)
        n121 = Unbundle By Name(w331) -> ("UI State"=w330:T14)
        n122 = case shown="\"Waiting for Exit\"" w330 {
          tunnel: w329 -> [_ _ w340 w345]
          tunnel: [w336 w337 w339 w343] -> w328
          tunnel: w327 -> [w336 w337 w338 w342]
          frame "Idle", Default {
          }
          frame "Acquiring and Logging" {
          }
          frame "Waiting for Exit" {
            n123 = call-poly "Enqueue Message.vi"("error in (no error)"=w338, "Message"="Verify Exit", "Message Queue"=w340) -> ("error out"=w339:errorcluster)  [unwired: 7 in, 1 out]
          }
          frame "Waiting for Stop" {
            n124 = call-poly "Enqueue Message.vi"("error in (no error)"=w342, "Message"="Verify Stop", "Message Queue"=w345) -> ("error out"=w343:errorcluster)  [unwired: 7 in, 1 out]
          }
        }
      }
      frame "Logging Stopped" {
        # "Logic for determining what action to take when the acquisition has stopped."
        n125 = Bundle By Name(cluster=w354, "Log On"=FALSE ("Acq On")) -> (w353:T3)
        n126 = Unbundle By Name(w353) -> ("UI State"=w352:T14)
        n127 = Unbundle By Name(w348) -> ("Record Ref"=w347:refnum<vi>)
        n128 = case shown="\"Acquiring and Logging\"" w352 {
          tunnel: w351 -> [_ _ w361 w366]
          tunnel: [w357 w358 w360 w364] -> w350
          tunnel: w349 -> [w357 w358 w359 w363]
          frame "Idle", Default {
          }
          frame "Acquiring and Logging" {
          }
          frame "Waiting for Exit" {
            n129 = call-poly "Enqueue Message.vi"("error in (no error)"=w359, "Message"="Verify Exit", "Message Queue"=w361) -> ("error out"=w360:errorcluster)  [unwired: 7 in, 1 out]
          }
          frame "Waiting for Stop" {
            n130 = call-poly "Enqueue Message.vi"("error in (no error)"=w363, "Message"="Verify Stop", "Message Queue"=w366) -> ("error out"=w364:errorcluster)  [unwired: 7 in, 1 out]
          }
        }
        n131 = property class="Bool"(reference=w347, "Value"=FALSE ("Start Saving")) -> ()  [unwired: 1 in, 2 out]
      }
      frame "Piezo Stopped" {
        # "Logic for determining what action to take when the acquisition has stopped."
        n132 = Bundle By Name(cluster=w372, "Piezo On"=FALSE ("Acq On")) -> (w371:T3)
        n133 = Unbundle By Name(w371) -> ("UI State"=w370:T14)
        n134 = case shown="\"Waiting for Exit\"" w370 {
          tunnel: w369 -> [_ _ w380 w385]
          tunnel: [w376 w377 w379 w383] -> w368
          tunnel: w367 -> [w376 w377 w378 w382]
          frame "Idle", Default {
          }
          frame "Acquiring and Logging" {
          }
          frame "Waiting for Exit" {
            n135 = call-poly "Enqueue Message.vi"("error in (no error)"=w378, "Message"="Verify Exit", "Message Queue"=w380) -> ("error out"=w379:errorcluster)  [unwired: 7 in, 1 out]
          }
          frame "Waiting for Stop" {
            n136 = call-poly "Enqueue Message.vi"("error in (no error)"=w382, "Message"="Verify Stop", "Message Queue"=w385) -> ("error out"=w383:errorcluster)  [unwired: 7 in, 1 out]
          }
        }
      }
      frame "XY Stopped" {
        # "Logic for determining what action to take when the acquisition has stopped."
        n137 = Bundle By Name(cluster=w391, "XY On"=FALSE ("Acq On")) -> (w390:T3)
        n138 = Unbundle By Name(w390) -> ("UI State"=w389:T14)
        n139 = case shown="\"Waiting for Stop\"" w389 {
          tunnel: w388 -> [_ _ w399 w404]
          tunnel: [w395 w396 w398 w402] -> w387
          tunnel: w386 -> [w395 w396 w397 w401]
          frame "Idle", Default {
          }
          frame "Acquiring and Logging" {
          }
          frame "Waiting for Exit" {
            n140 = call-poly "Enqueue Message.vi"("error in (no error)"=w397, "Message"="Verify Exit", "Message Queue"=w399) -> ("error out"=w398:errorcluster)  [unwired: 7 in, 1 out]
          }
          frame "Waiting for Stop" {
            n141 = call-poly "Enqueue Message.vi"("error in (no error)"=w401, "Message"="Verify Stop", "Message Queue"=w404) -> ("error out"=w402:errorcluster)  [unwired: 7 in, 1 out]
          }
        }
      }
      frame "Cap Stopped" {
        # "Logic for determining what action to take when the acquisition has stopped."
        n142 = Bundle By Name(cluster=w414, "Cap On"=FALSE ("Acq On")) -> (w413:T3)
        n143 = Unbundle By Name(w413) -> ("UI State"=w412:T14)
        n144 = control-ref of="Enable Sensor"() -> (w409:refnum<vi>)
        n145 = case shown="\"Idle\", Default" w412 {
          tunnel: w411 -> [_ _ w422 w427]
          tunnel: [w418 w419 w421 w425] -> w406
          tunnel: w410 -> [w418 w419 w420 w424]
          frame "Idle", Default {
          }
          frame "Acquiring and Logging" {
          }
          frame "Waiting for Exit" {
            n146 = call-poly "Enqueue Message.vi"("error in (no error)"=w420, "Message"="Verify Exit", "Message Queue"=w422) -> ("error out"=w421:errorcluster)  [unwired: 7 in, 1 out]
          }
          frame "Waiting for Stop" {
            n147 = call-poly "Enqueue Message.vi"("error in (no error)"=w424, "Message"="Verify Stop", "Message Queue"=w427) -> ("error out"=w425:errorcluster)  [unwired: 7 in, 1 out]
          }
        }
        n148 = property class="Bool (strict)"(reference=w409, "Value"=FALSE) -> (error out=w405:errorcluster)  [unwired: 1 in, 1 out]
        n149 = Merge Errors(w405, w406) -> (w407:errorcluster)
      }
      frame "Broadcast settings" {
        w437 = "Update Settings" ("Message")
        # "Display Data Source on the front panel"
        # "Send the 'Update Settings' message to the Logging and Acquisition message loops."
        n150 = Unbundle By Name(w431) -> ("Hardware Config"=w434:T9, "Logging Configuration"=w445:T6, "Capacitive Config"=w438:T8)
        n151 = Unbundle By Name(w434) -> ("Data Source"=w433:u16)
        n152 = call-poly "Enqueue Message.vi"("Message Data"=w434, "Message"=w437, "Message Queue"=w442) -> ("error out"=w446:errorcluster)  [unwired: 7 in, 1 out]
        n153 = case shown="1" w433 {
          tunnel: ["Counter (APD)" ("Message") "Analog in (photodiode)" ("Message")] -> w432
          frame 0, Default {
          }
          frame 1 {
          }
        }
        "Data Source" <- w432
        n154 = call-poly "Enqueue Message.vi"("error in (no error)"=w446, "Message Data"=w445, "Message"=w437, "Message Queue"=w441) -> ("error out"=w436:errorcluster)  [unwired: 6 in, 1 out]
        n155 = call-poly "Enqueue Message.vi"("error in (no error)"=w436, "Message Data"=w438, "Message"=w437, "Message Queue"=w439) -> ("error out"=w435:errorcluster)  [unwired: 6 in, 1 out]
        n156 = Unbundle By Name(w431) -> ("Hardware Config"=w430:T9)
        n157 = Unbundle By Name(w430) -> ("ADC Configuration"=w429:T11)
        n158 = Unbundle By Name(w429) -> ("Sample Rate (s/s)"=→"Sample Rate (s/s)":i32)
        n159 = Merge Errors(w435, w444) -> (w447:errorcluster)
      }
      frame "Launch Settings Dialog" {
        # "Launch the Settings Dialog when the user clicks the 'Settings' button."
        n160 = call "Settings Dialog.vi"("error in (no error)"=w457, "Settings in"=w458) -> ("error out"=w453:errorcluster, "Cancelled?"=w456:bool, "Settings out"=w454:T5)  [unwired: 6 in, 1 out]
        n161 = case shown="True" w456 {
          tunnel: w455 -> [w462 _]
          tunnel: w453 -> [w461 w463]
          tunnel: [w460 w463] -> w452
          frame False {
            n162 = call-poly "Enqueue Message.vi"("error in (no error)"=w461, "Message"="Broadcast Settings", "Message Queue"=w462) -> ("error out"=w460:errorcluster)  [unwired: 7 in, 1 out]
          }
          frame True {
          }
        }
      }
      frame "Error" {
        # "Error - Check the error message data and respond accordingly. This message is sent by the \"Error Handler\" VIs at the end of each loop in this application."
        n163 = Variant To Data(error in=w474, type=errorcluster {"status"=FALSE, "code"=0, "source"=""} ("error out"), Variant=w473) -> (data=w471:errorcluster, error out=w467:errorcluster)
        n164 = call <vilib>:"Simple Error Handler.vi"("error in (no error)"=w471) -> ()  [unwired: 4 in, 5 out]
        n165 = call-poly "Enqueue Message.vi"("Priority Message? (F)"=TRUE, "Message"="Exit", "Message Queue"=w470) -> ("error out"=w466:errorcluster)  [unwired: 7 in, 1 out]
        n166 = Merge Errors(w466, w467) -> (w465:errorcluster)
      }
      frame "Confirm Quit" {
        # "Confirm Quit - Message that can confirm whether or not the user wants to exit the application."
        n167 = Unbundle By Name(w478) -> ("UI State"=w477:T14)
        n168 = case shown="Default" w477 {
          tunnel: w482 -> [w489 w495]
          tunnel: w481 -> [w488 w493]
          tunnel: [w485 w492] -> w480
          tunnel: [T3 {"UI State"=enum."Idle", "Acq On"=FALSE, "Log On"=FALSE, "Piezo On"=FALSE, "XY On"=FALSE, "Cap On"=FALSE} ("UI State") w491] -> w479
          frame Default {
            # "If 'Confirm Quit' comes in while the system is idle, there is no need for a confirmation message."
            n169 = call-poly "Enqueue Message.vi"("Priority Message? (F)"=TRUE, "error in (no error)"=w488, "Message"="Exit", "Message Queue"=w489) -> ("error out"=w485:errorcluster)  [unwired: 6 in, 1 out]
          }
          frame "Acquiring and Logging" {
            n170 = Two Button Dialog(message="Are you sure you want to quit while the acquisition is running?" ("Confirm Quit Message"), 1:"No" ("No"), 2:"Yes" ("Yes")) -> (T button?=w494:bool)
            n171 = case shown="True" w494 {
              tunnel: w495 -> [_ w505]
              tunnel: w493 -> [w499 w504]
              tunnel: [w499 w503] -> w492
              tunnel: [T3 {"UI State"=enum."Idle", "Acq On"=FALSE, "Log On"=FALSE, "Piezo On"=FALSE, "XY On"=FALSE, "Cap On"=FALSE} ("UI State") T3 {"UI State"=enum."Idle", "Acq On"=FALSE, "Log On"=FALSE, "Piezo On"=FALSE, "XY On"=FALSE, "Cap On"=FALSE} ("UI State")] -> w491
              frame False {
                # "User did not want to quit."
              }
              frame True {
                n172 = call-poly "Enqueue Message.vi"("error in (no error)"=w504, "Message"="Stop", "Message Queue"=w505) -> ("error out"=w503:errorcluster)  [unwired: 7 in, 1 out]
              }
            }
          }
        }
      }
      frame "Exit" {
        # "Don't check the error outs. The acquisition and logging queues may have already been released."
        # "Close references owned by the Main VI."
        # "Stop the VI"
        # "Exit - Fire the User Event to stop the Event Handling Loop.  Also send Exit messages to the Acquisition and Logging loops."
        n173 = Release Queue(queue=w520, error in (no error)=w525) -> (error out=w517:errorcluster)  [unwired: 1 in, 2 out]
        n174 = call "Fire User Event - Stop.vi"("User Event - Stop"=w524) -> ("error out"=w523:errorcluster)  [unwired: 10 in]
        n175 = Release Queue(queue=w519, error in (no error)=w517) -> (error out=w515:errorcluster)  [unwired: 1 in, 2 out]
        n176 = Build Array(w513, w512, w511, w510, w509, w507, w506) -> (w508:refnum<queue>[])
        n177 = for {
          tunnel: w508 -> [w529] mode=indexing
          n178 = call-poly "Enqueue Message.vi"("Priority Message? (F)"=TRUE, "Message"="Exit", "Message Queue"=w529) -> ()  [unwired: 7 in, 2 out]
        }
        n179 = call "Release All Notifiers.vi"("error in (no error)"=w515, "All Data Notifiers"=w516) -> ("error out"=w514:errorcluster)  [unwired: 9 in]
        n180 = Merge Errors(w523, w514) -> (w526:errorcluster)
      }
      frame "---Copy This Frame---" {
        # "Duplicate this frame when creating new messages.  Change this comment in the duplicated frame to describe this message."
        n181 = Merge Errors(w535) -> (w534:errorcluster)
      }
      frame "Update Feedback Settings" {
        n182 = call-poly "Enqueue Message.vi"("error in (no error)"=w540, "Message Data"="Feedback Settings", "Message"="Update Feedback Settings", "Message Queue"=w538) -> ("error out"=w539:errorcluster)  [unwired: 6 in, 1 out]
      }
      frame "Start Feedback" {
        # "Tell Feedback Message Loop to go into feedback mode"
        n183 = control-ref of="Feedback Settings"() -> (w545:refnum<vi>)
        n184 = property class="Clust (strict)"(reference=w545) -> ("Value"=w544:T1)  [unwired: 1 in, 2 out]
        n185 = call-poly "Enqueue Message.vi"("error in (no error)"=w547, "Message Data"=w544, "Message"="Start Feedback", "Message Queue"=w548) -> ("error out"=w546:errorcluster)  [unwired: 6 in, 1 out]
        n186 = Merge Errors(w546) -> (w553:errorcluster)
      }
      frame "Stop Feedback" {
        # "Duplicate this frame when creating new messages.  Change this comment in the duplicated frame to describe this message."
        n187 = call-poly "Enqueue Message.vi"("error in (no error)"=w555, "Message"="Stop Feedback", "Message Queue"=w556) -> ("error out"=w554:errorcluster)  [unwired: 7 in, 1 out]
        n188 = Merge Errors(w554) -> (w561:errorcluster)
      }
      frame "Start Average and set" {
        # "Tell feedback loop to start averaging"
        # "Duplicate this frame when creating new messages.  Change this comment in the duplicated frame to describe this message."
        n189 = local read "Feedback Settings"() -> (w565:T1)
        n190 = Unbundle By Name(w565) -> ("Error Signal Source"=w564:u16)
        n191 = Bundle("Averaging Time (s)"="Averaging Time (s)", "Error Signal Source"=w564) -> (w562:T16)  [unwired: 1 in]
        n192 = call-poly "Enqueue Message.vi"("error in (no error)"=w567, "Message Data"=w562, "Message"="Start Average and set", "Message Queue"=w568) -> ("error out"=w566:errorcluster)  [unwired: 6 in, 1 out]
      }
      frame "Stop Average and set" {
        # "Duplicate this frame when creating new messages.  Change this comment in the duplicated frame to describe this message."
        n193 = call-poly "Enqueue Message.vi"("error in (no error)"=w574, "Message"="Stop Average and set", "Message Queue"=w575) -> ("error out"=w573:errorcluster)  [unwired: 7 in, 1 out]
        n194 = Merge Errors(w573) -> (w580:errorcluster)
      }
      frame "Adjust Setpoint" {
        # "Change the value of 'SETPOINT'"
        # "Duplicate this frame when creating new messages.  Change this comment in the duplicated frame to describe this message."
        n195 = Variant To Data(error in=w589, type=0.0 ("Running average"), Variant=w588) -> (data=w586:dbl, error out=w585:errorcluster)
        n196 = control-ref of="Setpoint (cnt)"() -> (w581:refnum<vi>)
        n197 = property class="DigNum (strict)"(reference=w581, error in=w585, "Val(Sgnl)"=w586) -> (error out=w584:errorcluster)  [unwired: 1 out]
        n198 = case shown="False" "Auto \nFB On" {
          tunnel: w584 -> [w593 w596]
          tunnel: [w593 w595] -> w583
          frame False {
          }
          frame True {
            # "'Press' the Enable feedback button"
            n199 = control-ref of="Enable Feedback!"() -> (w594:refnum<vi>)
            n200 = property class="Bool (strict)"(reference=w594, error in=w596, "Val(Sgnl)"=TRUE ("Value (Signaling)")) -> (error out=w595:errorcluster)  [unwired: 1 out]
          }
        }
      }
      frame "Start Logging" {
        # "Notify Logging Loop whether capactive is running or not"
        # "Start the logging loop"
        # "Duplicate this frame when creating new messages.  Change this comment in the duplicated frame to describe this message."
        n201 = control-ref of="Enable Sensor"() -> (w603:refnum<vi>)
        n202 = property class="Bool (strict)"(reference=w603) -> (error out=w602:errorcluster, "Value"=w601:bool)  [unwired: 1 in, 1 out]
        n203 = Bundle("Value"=w601, "Filename"="Filename", "Max. Samp"="Max. Samp") -> (w599:T17)  [unwired: 1 in]
        n204 = call-poly "Enqueue Message.vi"("error in (no error)"=w605, "Message Data"=w599, "Message"="Start", "Message Queue"=w606) -> ("error out"=w604:errorcluster)  [unwired: 6 in, 1 out]
        n205 = Merge Errors(w604, w602) -> (w611:errorcluster)
      }
      frame "Stop Logging" {
        # "Stop the logging loop"
        # "Duplicate this frame when creating new messages.  Change this comment in the duplicated frame to describe this message."
        n206 = call-poly "Enqueue Message.vi"("error in (no error)"=w613, "Message"="Stop", "Message Queue"=w614) -> ("error out"=w612:errorcluster)  [unwired: 7 in, 1 out]
        n207 = Merge Errors(w612) -> (w619:errorcluster)
      }
      frame "Log Default Name" {
        # "The logging loop tells the UI which directory it will save to, and what is the default file name (dataXXX) that is next in line"
        n208 = Variant To Data(error in=w624, type=cluster{"Save Path":path, "Save String":string} {"Save Path"=path "", "Save String"=""} ("output cluster"), Variant=w631) -> (data=w629:cluster{"Save Path":path, "Save String":string}, error out=w627:errorcluster)
        n209 = Unbundle(w629) -> ("Save Path"=w620:path, "Save String"=w628:string)
        n210 = control-ref of="Filename"() -> (w625:refnum<vi>)
        n211 = property on="Property Node" class="Str"(reference=w625, error in=w627, "Value"=w628) -> (error out=w626:errorcluster)  [unwired: 1 out]
        n212 = Equal?(x=path "", y=w620) -> (x = y?=w621:bool)
        n213 = Merge Errors(w626) -> (w630:errorcluster)
        n214 = case shown="False" w621 {
          tunnel: w620 -> [w635 _]
          frame False {
            # "update path unless empty"
            "Path" <- w635
          }
          frame True {
          }
        }
      }
      frame "Start Piezo Scan" {
        # "Duplicate this frame when creating new messages.  Change this comment in the duplicated frame to describe this message."
        n215 = call-poly "Enqueue Message.vi"("error in (no error)"=w640, "Message Data"="Scan Settings", "Message"="Start Scan", "Message Queue"=w637) -> ("error out"=w639:errorcluster)  [unwired: 6 in, 1 out]
        n216 = Merge Errors(w639) -> (w644:errorcluster)
      }
      frame "Launch Z Scan" {
        # "Run the Z-scan settings dialog, then tell the automation loop to run the z-scan with the settings determined by the dialog."
        n217 = local read "Filename"() -> (w645:string)
        n218 = call "Automation Settings Dialog.vi"("error in (no error)"=w649, "Filename"=w645) -> ("error out"=w648:errorcluster, "Cancelled?"=w646:bool, "Settings Out"=w647:T18)  [unwired: 7 in]
        n219 = case shown="False" w646 {
          tunnel: [w659 w661] -> w652
          tunnel: w650 -> [w658 _]
          tunnel: w648 -> [w657 w661]
          tunnel: w647 -> [w656 _]
          frame False {
            n220 = call-poly "Enqueue Message.vi"("error in (no error)"=w657, "Message Data"=w656, "Message"="Start z scan", "Message Queue"=w658) -> ("error out"=w659:errorcluster)  [unwired: 6 in, 1 out]
          }
          frame True {
          }
        }
        n221 = Merge Errors(w652) -> (w655:errorcluster)
      }
      frame "Abort Automation" {
        # "Duplicate this frame when creating new messages.  Change this comment in the duplicated frame to describe this message."
        n222 = call-poly "Enqueue Message.vi"("error in (no error)"=w665, "Message"="Abort", "Message Queue"=w662) -> ("error out"=w664:errorcluster)  [unwired: 7 in, 1 out]
        n223 = Merge Errors(w664) -> (w669:errorcluster)
      }
      frame "Stop Piezo Scan" {
        # "Duplicate this frame when creating new messages.  Change this comment in the duplicated frame to describe this message."
        n224 = call-poly "Enqueue Message.vi"("error in (no error)"=w672, "Message"="Stop Scan", "Message Queue"=w670) -> ("error out"=w671:errorcluster)  [unwired: 7 in, 1 out]
        n225 = Merge Errors(w671) -> (w677:errorcluster)
      }
      frame "Move Piezo" {
        # "Duplicate this frame when creating new messages.  Change this comment in the duplicated frame to describe this message."
        n226 = call-poly "Enqueue Message.vi"("error in (no error)"=w680, "Message Data"="Move to (um)", "Message"="Go To", "Message Queue"=w678) -> ("error out"=w679:errorcluster)  [unwired: 6 in, 1 out]
        n227 = Merge Errors(w679) -> (w686:errorcluster)
      }
      frame "Start XY" {
        # "Duplicate this frame when creating new messages.  Change this comment in the duplicated frame to describe this message."
        n228 = Unbundle By Name(w692) -> ("Enable Piezo"=w691:refnum<vi>)
        n229 = call-poly "Enqueue Message.vi"("error in (no error)"=w696, "Message"="Start", "Message Queue"=w694) -> ("error out"=w695:errorcluster)  [unwired: 7 in, 1 out]
        n230 = property class="Bool"(reference=w691, "DisabledEnum"=T15."Disabled and Grayed Out" ("Disabled")) -> (error out=w688:errorcluster)  [unwired: 1 in, 1 out]
        n231 = control-ref of="Jog Speed"() -> (w690:refnum<vi>)
        n232 = property class="Ring (strict)"(reference=w690, error in=w688, "Val(Sgnl)"=u16 0 ("Value (Signaling)")) -> (error out=w687:errorcluster)  [unwired: 1 out]
        n233 = Merge Errors(w687, w695) -> (w700:errorcluster)
      }
      frame "Stop XY" {
        # "Duplicate this frame when creating new messages.  Change this comment in the duplicated frame to describe this message."
        n234 = Unbundle By Name(w703) -> ("Enable Piezo"=w702:refnum<vi>)
        n235 = call-poly "Enqueue Message.vi"("error in (no error)"=w707, "Message"="Stop", "Message Queue"=w705) -> ("error out"=w706:errorcluster)  [unwired: 7 in, 1 out]
        n236 = property class="Bool"(reference=w702, "DisabledEnum"=T15."Enabled" ("Disabled")) -> (error out=w701:errorcluster)  [unwired: 1 in, 1 out]
        n237 = Merge Errors(w701, w706) -> (w711:errorcluster)
      }
      frame "Jog XY" {
        n238 = call-poly "Enqueue Message.vi"("error in (no error)"=w713, "Message Data"=w716, "Message"="Jog", "Message Queue"=w717) -> ("error out"=w712:errorcluster)  [unwired: 6 in, 1 out]
      }
      frame "Jog Speed" {
        n239 = call-poly "Enqueue Message.vi"("error in (no error)"=w722, "Message Data"=w723, "Message"="Speed", "Message Queue"=w724) -> ("error out"=w721:errorcluster)  [unwired: 6 in, 1 out]
      }
      frame "Start Cap" {
        # "Duplicate this frame when creating new messages.  Change this comment in the duplicated frame to describe this message."
        n240 = call-poly "Enqueue Message.vi"("error in (no error)"=w730, "Message"="Start", "Message Queue"=w728) -> ("error out"=w729:errorcluster)  [unwired: 7 in, 1 out]
        n241 = Merge Errors(w729) -> (w735:errorcluster)
      }
      frame "Stop Cap" {
        # "Duplicate this frame when creating new messages.  Change this comment in the duplicated frame to describe this message."
        n242 = call-poly "Enqueue Message.vi"("error in (no error)"=w738, "Message"="Stop", "Message Queue"=w736) -> ("error out"=w737:errorcluster)  [unwired: 7 in, 1 out]
        n243 = Merge Errors(w737) -> (w743:errorcluster)
      }
      frame "Enable Piezo" {
        # "Duplicate this frame when creating new messages.  Change this comment in the duplicated frame to describe this message."
        n244 = Unbundle By Name(w747) -> ("Enable XY Ref"=w746:refnum<vi>)
        n245 = call-poly "Enqueue Message.vi"("error in (no error)"=w750, "Message"="Start", "Message Queue"=w748) -> ("error out"=w749:errorcluster)  [unwired: 7 in, 1 out]
        n246 = property class="Bool"(reference=w746, "DisabledEnum"=T15."Disabled and Grayed Out" ("Disabled")) -> (error out=w744:errorcluster)  [unwired: 1 in, 1 out]
        n247 = Merge Errors(w744, w749) -> (w754:errorcluster)
      }
      frame "Disable Piezo" {
        # "Duplicate this frame when creating new messages.  Change this comment in the duplicated frame to describe this message."
        n248 = Unbundle By Name(w758) -> ("Enable XY Ref"=w757:refnum<vi>)
        n249 = call-poly "Enqueue Message.vi"("error in (no error)"=w761, "Message"="Stop", "Message Queue"=w759) -> ("error out"=w760:errorcluster)  [unwired: 7 in, 1 out]
        n250 = property class="Bool"(reference=w757, "DisabledEnum"=T15."Enabled" ("Disabled")) -> (error out=w755:errorcluster)  [unwired: 1 in, 1 out]
        n251 = Merge Errors(w755, w760) -> (w765:errorcluster)
      }
      frame "Verify Stop" {
        # "Duplicate this frame when creating new messages.  Change this comment in the duplicated frame to describe this message."
        n252 = Unbundle By Name(w774) -> ("Acq On"=w772:bool, "Log On"=w771:bool, "Piezo On"=w770:bool, "XY On"=w766:bool)
        n253 = Build Array(w772, w771, w770, w766) -> (w769:bool[])
        n254 = Or Array Elements(Boolean array=w769) -> (logical OR=w768:bool)
        n255 = Not(x=w768) -> (.not. x?=w767:bool)
        n256 = case shown="True" w767 {
          tunnel: [w779 w782] -> w776
          tunnel: w775 -> [w779 w781]
          tunnel: w773 -> [_ w780]
          frame False {
          }
          frame True {
            # "If everything is off, then update status."
            n257 = call-poly "Enqueue Message.vi"("error in (no error)"=w781, "Message Data"="Ready..." ("Message"), "Message"="Update Status", "Message Queue"=w780) -> ("error out"=w783:errorcluster)  [unwired: 6 in, 1 out]
            n258 = Merge Errors(w783) -> (w782:errorcluster)
          }
        }
      }
      frame "Verify Exit" {
        # "Duplicate this frame when creating new messages.  Change this comment in the duplicated frame to describe this message."
        n259 = Unbundle By Name(w794) -> ("Acq On"=w792:bool, "Log On"=w791:bool, "Piezo On"=w790:bool, "XY On"=w786:bool)
        n260 = Build Array(w792, w791, w790, w786) -> (w789:bool[])
        n261 = Or Array Elements(Boolean array=w789) -> (logical OR=w788:bool)
        n262 = Not(x=w788) -> (.not. x?=w787:bool)
        n263 = case shown="True" w787 {
          tunnel: [w799 w803] -> w796
          tunnel: w795 -> [w799 w802]
          tunnel: w793 -> [_ w801]
          frame False {
          }
          frame True {
            # "If everything is off, then exit."
            n264 = call-poly "Enqueue Message.vi"("Priority Message? (F)"=TRUE, "error in (no error)"=w802, "Message"="Exit", "Message Queue"=w801) -> ("error out"=w804:errorcluster)  [unwired: 6 in, 1 out]
            n265 = Merge Errors(w804) -> (w803:errorcluster)
          }
        }
      }
      frame Default {
        # "'Default' case only runs if there is a message that isn't defined in any of the other cases.  Output a programming error."
        n266 = xnode "Error Ring"("parameter 0"=w807) -> ("error out"=w808:errorcluster)
      }
    }
    n267 = call "Error Handler - Message Handling Loop.vi"("error in (no error)"=w51, "Message Queue"=w49) -> ("dup error in"=w50:errorcluster)  [unwired: 8 in, 1 out]
  }
  n268 = while {
    tunnel: w24 -> [w823]
    tunnel: [w818] -> w39
    shift-right: [w822] -> w32
    shift-left: w37 -> [w824]
    stop <- w821 stop-if-true
    # "Event Handling Loop"
    n269 = event shown="[5] \"Settings\": Value Change" {
      selector: w824 -> [_ _ _ _ _ _ _ _ _ _ _ _ _ _ _ _ _ _ _ _ _ _ _ _]
      dyn-events: [_ _ _ _ _ _ _ _ _ _ _ _ _ _ _ _ _ _ _ _ _ _ _ _] -> w822
      timeout: _ -> [_ _ _ _ _ _ _ _ _ _ _ _ _ _ _ _ _ _ _ _ _ _ _ _]
      tunnel: [_ _ _ _ _ _ _ _ _ _ _ _ _ _ _ _ _ _ _ _ _ _ TRUE ("Discard?") _] -> w821
      tunnel: w823 -> [w826 w831 w835 w842 w843 w845 w849 w853 w858 w866 w872 w883 w893 w905 w916 w922 w927 w933 w941 w950 w954 w959 w963 _]
      tunnel: [w828 w830 w833 w837 _ w847 w851 w855 w857 w865 w871 w882 w892 w903 w915 w921 w926 w932 w940 w947 w953 w962 _ _] -> w819
      tunnel: [w825 w829 w834 w838 w843 w844 w848 w852 w856 w864 _ _ _ _ _ _ _ w930 w939 w948 w952 w958 w963 _] -> w820
      event "Start": Value Change {
        n270 = event-data() -> ()  [unwired: 1 in, 1 out]
        n271 = call-poly "Enqueue Message.vi"("Message"="Start", "Message Queue"=w826) -> ("error out"=w828:errorcluster, "dup Message Queue"=w825:refnum<queue>)  [unwired: 8 in]
      }
      event "Stop": Value Change {
        n272 = event-data() -> ()  [unwired: 1 in, 1 out]
        n273 = call-poly "Enqueue Message.vi"("Message"="Stop", "Message Queue"=w831) -> ("error out"=w830:errorcluster, "dup Message Queue"=w829:refnum<queue>)  [unwired: 8 in]
      }
      event "Do move": Value Change {
        n274 = event-data() -> ()  [unwired: 1 in, 1 out]
        n275 = call-poly "Enqueue Message.vi"("Message"="Move Piezo", "Message Queue"=w835) -> ("error out"=w833:errorcluster, "dup Message Queue"=w834:refnum<queue>)  [unwired: 8 in]
      }
      event Panel Close? {
        # "Send the 'Confirm Quit' message if the user closes the panel of the VI. Discard the event so the 'Confirm Quit' message has a chance to run."
        n276 = event-data() -> ()  [unwired: 1 in, 1 out]
        n277 = call-poly "Enqueue Message.vi"("Priority Message? (F)"=TRUE, "Message"="Confirm Quit", "Message Queue"=w842) -> ("error out"=w837:errorcluster, "dup Message Queue"=w838:refnum<queue>)  [unwired: 7 in]
        n278 = event-data("Discard?"=TRUE) -> ()  [unwired: 1 in, 1 out]
      }
      event Application Instance Close {
        n279 = event-data() -> ()  [unwired: 1 in, 1 out]
      }
      event "Settings": Value Change {
        n280 = event-data() -> ()  [unwired: 1 in, 1 out]
        n281 = call-poly "Enqueue Message.vi"("Message"="Launch Settings Dialog", "Message Queue"=w845) -> ("error out"=w847:errorcluster, "dup Message Queue"=w844:refnum<queue>)  [unwired: 8 in]
      }
      event "Start Z scan": Value Change {
        n282 = event-data() -> ()  [unwired: 1 in, 1 out]
        n283 = call-poly "Enqueue Message.vi"("Message"="Launch Z Scan", "Message Queue"=w849) -> ("error out"=w851:errorcluster, "dup Message Queue"=w848:refnum<queue>)  [unwired: 8 in]
      }
      event "Abort": Value Change {
        n284 = event-data() -> ()  [unwired: 1 in, 1 out]
        n285 = call-poly "Enqueue Message.vi"("Message"="Abort Automation", "Message Queue"=w853) -> ("error out"=w855:errorcluster, "dup Message Queue"=w852:refnum<queue>)  [unwired: 8 in]
      }
      event "Start Saving": Value Change {
        n286 = event-data() -> ()  [unwired: 1 in, 1 out]
        n287 = case shown="True" "Start Saving" {
          tunnel: ["Stop Logging" ("Message") "Start Logging" ("Message")] -> w859
          frame False {
          }
          frame True {
          }
        }
        n288 = call-poly "Enqueue Message.vi"("Message"=w859, "Message Queue"=w858) -> ("error out"=w857:errorcluster, "dup Message Queue"=w856:refnum<queue>)  [unwired: 8 in]
      }
      event "Enable Piezo": Value Change {
        n289 = event-data() -> ()  [unwired: 1 in, 1 out]
        n290 = case shown="True" "Enable Piezo" {
          tunnel: ["Disable Piezo" ("Message") "Enable Piezo" ("Message")] -> w867
          frame False {
          }
          frame True {
          }
        }
        n291 = call-poly "Enqueue Message.vi"("Message"=w867, "Message Queue"=w866) -> ("error out"=w865:errorcluster, "dup Message Queue"=w864:refnum<queue>)  [unwired: 8 in]
      }
      event "Previous Button": Value Change {
        n292 = event-data() -> ("NewVal"=w870:bool)  [unwired: 1 in]
        n293 = case shown="False" w870 {
          tunnel: w872 -> [w875 w879]
          tunnel: [w873 w877] -> w871
          frame True {
            n294 = call-poly "Enqueue Message.vi"("Message Data"="Left" ("Message"), "Message"="Jog XY", "Message Queue"=w875) -> ("error out"=w873:errorcluster)  [unwired: 7 in, 1 out]
          }
          frame False {
            n295 = call-poly "Enqueue Message.vi"("Message Data"="Stop" ("Message"), "Message"="Jog XY", "Message Queue"=w879) -> ("error out"=w877:errorcluster)  [unwired: 7 in, 1 out]
          }
        }
      }
      event "Next Button": Value Change {
        n296 = event-data() -> ()  [unwired: 1 in, 1 out]
        n297 = case shown="False" "Next Button" {
          tunnel: w883 -> [w886 w890]
          tunnel: [w884 w888] -> w882
          frame True {
            n298 = call-poly "Enqueue Message.vi"("Message Data"="Right" ("Message"), "Message"="Jog XY", "Message Queue"=w886) -> ("error out"=w884:errorcluster)  [unwired: 7 in, 1 out]
          }
          frame False {
            n299 = call-poly "Enqueue Message.vi"("Message Data"="Stop" ("Message"), "Message"="Jog XY", "Message Queue"=w890) -> ("error out"=w888:errorcluster)  [unwired: 7 in, 1 out]
          }
        }
      }
      event "Up Button": Value Change {
        n300 = event-data() -> ("NewVal"=w894:bool)  [unwired: 1 in]
        n301 = case shown="False" w894 {
          tunnel: w893 -> [w897 w901]
          tunnel: [w895 w899] -> w892
          frame True {
            n302 = call-poly "Enqueue Message.vi"("Message Data"="Up" ("Message"), "Message"="Jog XY", "Message Queue"=w897) -> ("error out"=w895:errorcluster)  [unwired: 7 in, 1 out]
          }
          frame False {
            n303 = call-poly "Enqueue Message.vi"("Message Data"="Stop" ("Message"), "Message"="Jog XY", "Message Queue"=w901) -> ("error out"=w899:errorcluster)  [unwired: 7 in, 1 out]
          }
        }
      }
      event "Down Button": Value Change {
        n304 = event-data() -> ("NewVal"=w904:bool)  [unwired: 1 in]
        n305 = case shown="True" w904 {
          tunnel: w905 -> [w908 w912]
          tunnel: [w906 w910] -> w903
          frame True {
            n306 = call-poly "Enqueue Message.vi"("Message Data"="Down" ("Message"), "Message"="Jog XY", "Message Queue"=w908) -> ("error out"=w906:errorcluster)  [unwired: 7 in, 1 out]
          }
          frame False {
            n307 = call-poly "Enqueue Message.vi"("Message Data"="Stop" ("Message"), "Message"="Jog XY", "Message Queue"=w912) -> ("error out"=w910:errorcluster)  [unwired: 7 in, 1 out]
          }
        }
      }
      event "Enable XY": Value Change {
        n308 = event-data() -> ()  [unwired: 1 in, 1 out]
        n309 = case shown="False" "Enable XY" {
          tunnel: ["Stop XY" ("Message") "Start XY" ("Message")] -> w917
          frame False {
          }
          frame True {
          }
        }
        n310 = call-poly "Enqueue Message.vi"("Message"=w917, "Message Queue"=w916) -> ("error out"=w915:errorcluster)  [unwired: 8 in, 1 out]
      }
      event "Enable Sensor": Value Change {
        n311 = event-data() -> ()  [unwired: 1 in, 1 out]
        n312 = case shown="False" "Enable Sensor" {
          tunnel: ["Stop Cap" ("Message") "Start Cap" ("Message")] -> w923
          frame False {
          }
          frame True {
          }
        }
        n313 = call-poly "Enqueue Message.vi"("Message"=w923, "Message Queue"=w922) -> ("error out"=w921:errorcluster)  [unwired: 8 in, 1 out]
      }
      event "Jog Speed": Value Change {
        n314 = event-data() -> ()  [unwired: 1 in, 1 out]
        n315 = call-poly "Enqueue Message.vi"("Message Data"="Jog Speed", "Message"="Jog Speed", "Message Queue"=w927) -> ("error out"=w926:errorcluster)  [unwired: 7 in, 1 out]
      }
      event "Enable Feedback!": Value Change {
        n316 = event-data() -> ()  [unwired: 1 in, 1 out]
        n317 = case shown="False" "Enable Feedback!" {
          tunnel: ["Stop Feedback" ("Message") "Start Feedback" ("Message")] -> w934
          frame False {
          }
          frame True {
          }
        }
        n318 = call-poly "Enqueue Message.vi"("Message"=w934, "Message Queue"=w933) -> ("error out"=w932:errorcluster, "dup Message Queue"=w930:refnum<queue>)  [unwired: 8 in]
      }
      event "Scan!": Value Change {
        n319 = event-data() -> ()  [unwired: 1 in, 1 out]
        n320 = case shown="False" "Scan!" {
          tunnel: ["Stop Piezo Scan" ("Message") "Start Piezo Scan" ("Message")] -> w942
          tunnel: [FALSE ("Priority Message? (F)") FALSE ("Priority Message? (F)")] -> w937
          frame False {
          }
          frame True {
          }
        }
        n321 = call-poly "Enqueue Message.vi"("Priority Message? (F)"=w937, "Message"=w942, "Message Queue"=w941) -> ("error out"=w940:errorcluster, "dup Message Queue"=w939:refnum<queue>)  [unwired: 7 in]
      }
      event "Feedback Settings": Value Change {
        n322 = event-data() -> ()  [unwired: 1 in, 1 out]
        n323 = call-poly "Enqueue Message.vi"("Message"="Update Feedback Settings", "Message Queue"=w950) -> ("error out"=w947:errorcluster, "dup Message Queue"=w948:refnum<queue>)  [unwired: 8 in]
      }
      event "Average and send\nto Setpoint": Value Change {
        n324 = event-data() -> ()  [unwired: 1 in, 1 out]
        n325 = case shown="False" "Average and send\nto Setpoint" {
          tunnel: ["Stop Average and set" ("Message") "Start Average and set" ("Message")] -> w955
          frame False {
          }
          frame True {
          }
        }
        n326 = call-poly "Enqueue Message.vi"("Message"=w955, "Message Queue"=w954) -> ("error out"=w953:errorcluster, "dup Message Queue"=w952:refnum<queue>)  [unwired: 8 in]
      }
      event "Exit": Value Change; Panel Close {
        w960 = TRUE  # Priority Message
        # "The UI Message Loop handles sending the Exit message to other loops."
        n327 = event-data() -> ()  [unwired: 1 in, 1 out]
        n328 = call-poly "Enqueue Message.vi"("Priority Message? (F)"=w960, "Message"="Exit", "Message Queue"=w959) -> ("error out"=w962:errorcluster, "dup Message Queue"=w958:refnum<queue>)  [unwired: 7 in]
      }
      event User Event {
        # "The Message Handling Loop processed an \"Exit\" message, which fired this event to stop the Event Handling Loop."
        n329 = event-data() -> ()  [unwired: 1 in, 1 out]
        n330 = local write "Status"("Exit" ("Exit String")) -> ()
      }
      event "Scan Settings": Value Change {
        n331 = event-data() -> ()  [unwired: 1 in, 1 out]
        n332 = local read "Scan Settings"() -> (w974:T2)
        n333 = Unbundle By Name(w974) -> ("Dwell Time (s)"=w967:dbl, "Max Height"=w973:dbl, "Min Height"=w972:dbl, "Step Size (um)"=w970:dbl)
        n334 = Subtract(x=w973, y=w972) -> (x-y=w971:dbl)
        n335 = Divide(x=w971, y=w970) -> (x/y=w969:dbl)
        n336 = Round Toward -Infinity(1:w969) -> (0:w968:dbl)
        n337 = Multiply(x=w967, y=w968) -> (x*y=→"Scan Duration: (s)":dbl)
      }
    }
    n338 = call "Error Handler - Event Handling Loop.vi"("error in (no error)"=w819, "Message Queue"=w820) -> ("dup error in"=w818:errorcluster)  [unwired: 8 in, 1 out]
  }
  n339 = while {
    tunnel: w18 -> [w977]
    stop <- w978 stop-if-true
    n340 = Wait on Notification(notifier=w977) -> (notification=w979:T19, error out=w978:errorcluster)  [unwired: 3 in, 2 out]
    n341 = Unbundle By Name(w979) -> ("X Position"=→"X":sgl, "Y Position"=→"Y":sgl)
  }
  n342 = while "Data Display Loop" {
    tunnel: w20 -> [w998]
    stop <- w1004 stop-if-true
    # "Data Display Loop"
    n343 = local read "Sample Rate (s/s)"() -> (w993:i32)
    n344 = Wait on Notification(notifier=w998) -> (notification=w997:T20, error out=w1004:errorcluster)  [unwired: 3 in, 2 out]
    n345 = Unbundle By Name(w997) -> ("data"=w990:dbl[][], "t0"=w987:i32)
    n346 = Reciprocal(x=w993) -> (1/x=w986:dbl)
    n347 = Multiply(x=w987, y=w986) -> (x*y=w988:dbl)
    n348 = To Time Stamp(1:w988) -> (0:w989:timestamp)
    n349 = for {
      tunnel: w990 -> [w1008] mode=indexing
      tunnel: w986 -> [w1007]
      tunnel: [w1006] -> w983 mode=indexing
      tunnel: w989 -> [w1005]
      n350 = Bundle By Name("Y"=w1008, "dt"=w1007, "t0"=w1005) -> (w1006:waveform(dbl))  [unwired: 1 in]
    }
    n351 = Index Array(array=w983, index="Blue") -> (element=w984:waveform(dbl))
    n352 = Array Subset(array=w983, index=0 ("index (row)"), length=3) -> (→"Waveform Chart":waveform(dbl)[])
    n353 = Index Array(array=w983, index="Red") -> (element=w981:waveform(dbl))
    n354 = Build Array(w984, w981) -> (→"Data":waveform(dbl)[])
    n355 = Index Array(array=w990, index (row)="Channel") -> (element=w996:dbl[])  [unwired: 1 in]
    n356 = for {
      tunnel: w996 -> [w1024] mode=indexing
      tunnel: "PSD points" -> [w1017]
      tunnel: w993 -> [w1013]
      # "add binning here to show \nbinned PSD in real time"
      n357 = call <vilib>:"Power Spectrum PtByPt.vi"("initialize"="initialize", "sample length"=w1017, "x"=w1024) -> ("Power Spectrum"=w1019:dbl[])  [unwired: 1 in, 1 out]
      n358 = Divide(x=w1013, y=w1017) -> (x/y=w1021:dbl)
      n359 = Divide(x=w1017, y=2.0) -> (x/y=w1016:dbl)
      n360 = Increment(x=w1016) -> (x+1=w1015:dbl)
      n361 = Array Subset(array=w1019, length=w1015) -> (w1014:dbl[])  [unwired: 1 in]
      n362 = Bundle("t"=0.0, w1021, w1014) -> (→"PSD":cluster{"t":dbl, dbl, dbl[]})  [unwired: 1 in]
    }
    n363 = call-poly <vilib>:"Averaged DC-RMS.vi"("averaging time"=1000.0, "averaging type"=enum16{"Linear", "Exponential"}."Linear", "signal in"=w996) -> ("RMS value waveform"=w1001:waveform(dbl), "data ready"=w1000:bool)  [unwired: 4 in, 3 out]
    n364 = case shown="True" w1000 {
      tunnel: w1001 -> [_ w1012]
      frame False {
      }
      frame True {
        n365 = Unbundle By Name(w1012) -> ("Y"=w1011:dbl[])
        n366 = Index Array(array=w1011, index=0) -> (element=→"average":dbl)
      }
    }
  }
  n367 = while {
    tunnel: w19 -> [w1026]
    stop <- w1025 stop-if-true
    n368 = Wait on Notification(notifier=w1026) -> (notification=w1028:T21, error out=w1025:errorcluster)  [unwired: 3 in, 2 out]
    n369 = Unbundle By Name(w1028) -> ("PiezoPosition"=→"PiezoPosition":sgl)
  }
  n370 = while {
    tunnel: w6 -> [w1038]
    stop <- w1039 stop-if-true
    n371 = Wait on Notification(notifier=w1038) -> (notification=w1034:T22, error out=w1039:errorcluster)  [unwired: 3 in, 2 out]
    n372 = Unbundle By Name(w1034) -> ("Error signal"=w1033:dbl[], "Setpoint"=w1031:dbl, "Last average"=→"Waveform Chart 2":dbl)
    n373 = Index Array(array=w1033, index=0) -> (element=w1032:dbl)
    n374 = Subtract(x=w1032, y=w1031) -> (x-y=w1030:dbl)
    n375 = Multiply(x=1000.0, y=w1030) -> (x*y=→"Error" →"mean":dbl)
  }
  n376 = while {
    tunnel: w9 -> [w1042]
    stop <- w1043 stop-if-true
    n377 = Wait on Notification(notifier=w1042) -> (notification=w1041:T23, error out=w1043:errorcluster)  [unwired: 3 in, 2 out]
    n378 = Unbundle By Name(w1041) -> ("Readout"=→"Cap Readout":sgl)  [unwired: 1 out]
  }
  n379 = Unregister For Events(event registration refnum=w32, error in=w39) -> (error out=w33:errorcluster)
  n380 = property on="Data" class="WFChart (strict)"("History Data"=waveform(dbl)[][] []) -> ()  [unwired: 2 in, 2 out]
  n381 = property on="Waveform Chart" class="WFChart (strict)"("History Data"=waveform(dbl)[][] []) -> ()  [unwired: 2 in, 2 out]
  n382 = Merge Errors(w33, w40, w10) -> (w38:errorcluster)
  n383 = call "Destroy User Event - Stop.vi"("error in (no error)"=w38, "User Event - Stop"=w36) -> ("error out"=w26:errorcluster)  [unwired: 9 in]
  n384 = disable-structure shown="Default" {
    disable-tunnel: w26 -> [_ _]
    frame condition #0 {
      # "Call Quit LabVIEW if running as a built application."
      n385 = Quit LabVIEW() -> ()  [unwired: 1 in]
    }
    frame condition #1 (active) {
    }
  }
